vi "Coral Controller.vi"(3 "error in":errorcluster) -> ()   [LabVIEW 2023]
doc: "This VI executes continuously carrying out the current operation and responding to updates or new operations. It will often contain the timing or control code that is difficult to place directly in TeleOp. This VI generally opens all sensors and motors and isolates the rest of the robot code from knowing how the operations are carried out."
uses:
  <vilib>/Rock Robotics/WPI/Framework/Completion Status.ctl
  Coral Setpoints.ctl
  Coral Operations.ctl
  Support Code/Teleop Util/Coral States.ctl
  Support Code/Teleop Util/Scoring Levels.ctl
  <vilib>/Rock Robotics/WPI/ThirdParty/REV Robotics/REVLib/Typedef/Spark MAX Idle Mode.ctl
  <vilib>/Rock Robotics/WPI/ThirdParty/REV Robotics/REVLib/Typedef/SPARK Closed Loop Slot.ctl
  <vilib>/Rock Robotics/SystemInterfaces/DIO/FPGA_DIOChannel.ctl
  <vilib>/Rock Robotics/WPI/ThirdParty/REV Robotics/REVLib/Typedef/Spark MAX Control Type.ctl
  <vilib>/Rock Robotics/WPI/ThirdParty/REV Robotics/REVLib/SubVI/Public/SPARK Open Brushless.vi
  <vilib>/Rock Robotics/WPI/ThirdParty/REV Robotics/REVLib/SubVI/Public/SPARK Configure Basic Idle Mode.vi
  <vilib>/Rock Robotics/WPI/ThirdParty/REV Robotics/REVLib/SubVI/Public/SPARK Configure Basic Inverted.vi
  <vilib>/Rock Robotics/WPI/ThirdParty/REV Robotics/REVLib/SubVI/Public/SPARK Configure Encoder Conversion Factors.vi
  <vilib>/Rock Robotics/WPI/ThirdParty/REV Robotics/REVLib/SubVI/Public/SPARK Configure Limit Switch Reverse.vi
  <vilib>/Rock Robotics/WPI/ThirdParty/REV Robotics/REVLib/SubVI/Public/SPARK Configure Soft Limit Forward.vi
  <vilib>/Rock Robotics/WPI/ThirdParty/REV Robotics/REVLib/SubVI/Public/SPARK Configure Soft Limit Reverse.vi
  <vilib>/Rock Robotics/WPI/ThirdParty/REV Robotics/REVLib/SubVI/Public/SPARK Configure Power Smart Current Limit.vi
  <vilib>/Rock Robotics/WPI/ThirdParty/REV Robotics/REVLib/SubVI/Public/SPARK Configure Closed Loop Miscellaneous.vi
  <vilib>/Rock Robotics/Network Tables/NT Write String.vi
  Framework/Robot Global Data.vi
  <vilib>/Rock Robotics/Network Tables/NT Read Number.vi
  <vilib>/Rock Robotics/WPI/ThirdParty/REV Robotics/REVLib/SubVI/Public/SPARK Get Encoder Status Position.vi
  <vilib>/Rock Robotics/WPI/ThirdParty/REV Robotics/REVLib/SubVI/Public/SPARK Get Device Status Output Current.vi
  <vilib>/Rock Robotics/WPI/ThirdParty/REV Robotics/REVLib/SubVI/Public/SPARK Get Encoder Status Velocity.vi
  <vilib>/Rock Robotics/Network Tables/NT Write Number.vi
  <vilib>/Rock Robotics/WPI/ThirdParty/REV Robotics/REVLib/Typedef/Spark MAX Limit Switch Polarity.ctl
  <vilib>/Rock Robotics/WPI/ThirdParty/REV Robotics/REVLib/SubVI/Public/SPARK Configure Follower Mode From Ref.vi
  <vilib>/Rock Robotics/WPI/ThirdParty/REV Robotics/REVLib/SubVI/Public/SPARK Configure Limit Switch Forward.vi
  <vilib>/Rock Robotics/Network Tables/NT Write Boolean.vi
panel:
  out "Coral Seen":dbl(graph)
  out "Detect DIO2?":bool
  out "Detect DIO1?":bool
  in  "Arbitrary Feed Forward (0)":dbl=0.7
  out "End Time":dbl=1.16
  out "Current":dbl(graph)=8.571428571428571
  in  "Trapezoid Fly off?":bool
  out "Grounded Trapezoid":cluster{"Sensor Velocity":dbl, "Numeric":dbl}[](graph)=[{"Sensor Velocity"=-0.8645192980766296, "Numeric"=0.0}, {"Sensor Velocity"=-0.6395611763000488, "Numeric"=130.0}, {"Sensor Velocity"=0.6042479872703552, "Numeric"=260.0}, {"Sensor Velocity"=9.457396507263184, "Numeric"=390.0}, {"Sensor Velocity"=42.07109451293945, "Numeric"=520.0}, {"Sensor Velocity"=110.76964569091797, "Numeric"=650.0}, {"Sensor Velocity"=199.5862579345703, "Numeric"=780.0}, {"Sensor Velocity"=314.9165344238281, "Numeric"=910.0000000000001}, {"Sensor Velocity"=458.24102783203125, "Numeric"=1040.0}, {"Sensor Velocity"=610.0145263671875, "Numeric"=1170.0}, {"Sensor Velocity"=743.2603759765625, "Numeric"=1300.0}, {"Sensor Velocity"=877.9422607421875, "Numeric"=1430.0}, {"Sensor Velocity"=1007.7548828125, "Numeric"=1560.0}, {"Sensor Velocity"=1120.9271240234375, "Numeric"=1690.0}, {"Sensor Velocity"=1236.4169921875, "Numeric"=1820.0000000000002}, {"Sensor Velocity"=1353.0106201171875, "Numeric"=1950.0}, {"Sensor Velocity"=1475.4154052734375, "Numeric"=2080.0}, {"Sensor Velocity"=1603.7957763671875, "Numeric"=2210.0}, {"Sensor Velocity"=1739.5540771484375, "Numeric"=2340.0}, {"Sensor Velocity"=1868.9521484375, "Numeric"=2470.0}, {"Sensor Velocity"=1992.354736328125, "Numeric"=2600.0}, {"Sensor Velocity"=2117.319091796875, "Numeric"=2730.0}, {"Sensor Velocity"=2234.47900390625, "Numeric"=2860.0}, {"Sensor Velocity"=2350.825439453125, "Numeric"=2990.0}, {"Sensor Velocity"=2471.163818359375, "Numeric"=3120.0}, {"Sensor Velocity"=2591.919189453125, "Numeric"=3250.0}, {"Sensor Velocity"=2712.11083984375, "Numeric"=3380.0}, {"Sensor Velocity"=2833.210205078125, "Numeric"=3510.0000000000005}, {"Sensor Velocity"=2956.64697265625, "Numeric"=3640.0000000000005}, {"Sensor Velocity"=3072.224365234375, "Numeric"=3769.9999999999995}, {"Sensor Velocity"=3190.86376953125, "Numeric"=3810.188567638397}, {"Sensor Velocity"=3313.081298828125, "Numeric"=3680.188567638397}, {"Sensor Velocity"=3434.365234375, "Numeric"=3550.188567638397}, {"Sensor Velocity"=3542.049560546875, "Numeric"=3420.188567638397}, {"Sensor Velocity"=3607.70849609375, "Numeric"=3290.1885676383968}, {"Sensor Velocity"=3606.5849609375, "Numeric"=3160.1885676383977}, {"Sensor Velocity"=3526.638427734375, "Numeric"=3030.188567638397}, {"Sensor Velocity"=3369.229248046875, "Numeric"=2900.188567638397}, {"Sensor Velocity"=3153.94970703125, "Numeric"=2770.188567638397}, {"Sensor Velocity"=2924.535400390625, "Numeric"=2640.188567638397}, {"Sensor Velocity"=2719.2861328125, "Numeric"=2510.188567638397}, {"Sensor Velocity"=2555.581787109375, "Numeric"=2380.188567638397}, {"Sensor Velocity"=2438.929443359375, "Numeric"=2250.188567638397}, {"Sensor Velocity"=2356.54638671875, "Numeric"=2120.188567638397}, {"Sensor Velocity"=2284.232666015625, "Numeric"=1990.1885676383972}, {"Sensor Velocity"=2199.458740234375, "Numeric"=1860.188567638397}, {"Sensor Velocity"=2090.252197265625, "Numeric"=1730.1885676383968}, {"Sensor Velocity"=1953.88427734375, "Numeric"=1600.1885676383977}, {"Sensor Velocity"=1794.5289306640625, "Numeric"=1470.1885676383977}, {"Sensor Velocity"=1637.5787353515625, "Numeric"=1340.1885676383972}, {"Sensor Velocity"=1485.1500244140625, "Numeric"=1210.1885676383972}, {"Sensor Velocity"=1346.7877197265625, "Numeric"=1080.1885676383972}, {"Sensor Velocity"=1225.3587646484375, "Numeric"=950.1885676383968}, {"Sensor Velocity"=1115.109619140625, "Numeric"=820.1885676383968}, {"Sensor Velocity"=999.061279296875, "Numeric"=690.1885676383968}, {"Sensor Velocity"=821.3626708984375, "Numeric"=560.1885676383968}, {"Sensor Velocity"=596.3208618164062, "Numeric"=430.1885676383963}, {"Sensor Velocity"=392.0470886230469, "Numeric"=300.18856763839767}, {"Sensor Velocity"=209.99317932128906, "Numeric"=170.18856763839767}, {"Sensor Velocity"=60.287471771240234, "Numeric"=0.0}, {"Sensor Velocity"=-4.871912956237793, "Numeric"=0.0}]
  out "Sensor Experiment":bool
  out "Post-Trapezoid Sensor Position":dbl=-34.25307083129883
  out "Scoring Sequence Trapezoid":cluster{"Sensor Velocity":dbl, "Numeric":dbl}[](graph)=[{"Sensor Velocity"=0.0, "Numeric"=-0.0}, {"Sensor Velocity"=0.0026157922111451626, "Numeric"=-130.0}, {"Sensor Velocity"=-2.9558451175689697, "Numeric"=-260.0}, {"Sensor Velocity"=-16.448101043701172, "Numeric"=-390.0}, {"Sensor Velocity"=-48.15019607543945, "Numeric"=-520.0}, {"Sensor Velocity"=-107.9851303100586, "Numeric"=-650.0}, {"Sensor Velocity"=-196.86322021484375, "Numeric"=-780.0}, {"Sensor Velocity"=-303.8765869140625, "Numeric"=-910.0000000000001}, {"Sensor Velocity"=-431.81890869140625, "Numeric"=-1040.0}, {"Sensor Velocity"=-570.7528076171875, "Numeric"=-1170.0}, {"Sensor Velocity"=-702.0759887695312, "Numeric"=-1300.0}, {"Sensor Velocity"=-836.3681640625, "Numeric"=-1430.0}, {"Sensor Velocity"=-966.5980224609375, "Numeric"=-1560.0}, {"Sensor Velocity"=-1093.2154541015625, "Numeric"=-1690.0}, {"Sensor Velocity"=-1219.048095703125, "Numeric"=-1820.0000000000002}, {"Sensor Velocity"=-1337.7606201171875, "Numeric"=-1950.0}, {"Sensor Velocity"=-1451.64306640625, "Numeric"=-2080.0}, {"Sensor Velocity"=-1571.863525390625, "Numeric"=-2210.0}, {"Sensor Velocity"=-1691.6943359375, "Numeric"=-2340.0}, {"Sensor Velocity"=-1812.6131591796875, "Numeric"=-2470.0}, {"Sensor Velocity"=-1932.349853515625, "Numeric"=-2600.0}, {"Sensor Velocity"=-2050.272216796875, "Numeric"=-2730.0}, {"Sensor Velocity"=-2164.339111328125, "Numeric"=-2860.0}, {"Sensor Velocity"=-2275.850341796875, "Numeric"=-2990.0}, {"Sensor Velocity"=-2386.736328125, "Numeric"=-3120.0}, {"Sensor Velocity"=-2496.785400390625, "Numeric"=-3250.0}, {"Sensor Velocity"=-2606.660400390625, "Numeric"=-3380.0}, {"Sensor Velocity"=-2717.8173828125, "Numeric"=-3510.0000000000005}, {"Sensor Velocity"=-2827.43994140625, "Numeric"=-3640.0000000000005}, {"Sensor Velocity"=-2936.3876953125, "Numeric"=-3769.9999999999995}, {"Sensor Velocity"=-3045.58251953125, "Numeric"=-3845.9956407546997}, {"Sensor Velocity"=-3152.45458984375, "Numeric"=-3715.9956407546997}, {"Sensor Velocity"=-3255.081298828125, "Numeric"=-3585.9956407546997}, {"Sensor Velocity"=-3346.31103515625, "Numeric"=-3455.9956407546997}, {"Sensor Velocity"=-3405.5927734375, "Numeric"=-3325.9956407546993}, {"Sensor Velocity"=-3413.553955078125, "Numeric"=-3195.9956407547}, {"Sensor Velocity"=-3357.670166015625, "Numeric"=-3065.9956407546997}, {"Sensor Velocity"=-3238.325927734375, "Numeric"=-2935.9956407546997}, {"Sensor Velocity"=-3070.0546875, "Numeric"=-2805.9956407546997}, {"Sensor Velocity"=-2879.5595703125, "Numeric"=-2675.9956407546997}, {"Sensor Velocity"=-2695.614501953125, "Numeric"=-2545.9956407546997}, {"Sensor Velocity"=-2537.822021484375, "Numeric"=-2415.9956407546997}, {"Sensor Velocity"=-2411.872802734375, "Numeric"=-2285.9956407546997}, {"Sensor Velocity"=-2310.73583984375, "Numeric"=-2155.9956407546997}, {"Sensor Velocity"=-2222.242431640625, "Numeric"=-2025.9956407546997}, {"Sensor Velocity"=-2135.021484375, "Numeric"=-1895.9956407546995}, {"Sensor Velocity"=-2037.541259765625, "Numeric"=-1765.9956407546993}, {"Sensor Velocity"=-1922.8583984375, "Numeric"=-1635.9956407547002}, {"Sensor Velocity"=-1792.849609375, "Numeric"=-1505.9956407547002}, {"Sensor Velocity"=-1655.527099609375, "Numeric"=-1375.9956407546997}, {"Sensor Velocity"=-1512.610595703125, "Numeric"=-1245.9956407546997}, {"Sensor Velocity"=-1377.0655517578125, "Numeric"=-1115.9956407546997}, {"Sensor Velocity"=-1248.7752685546875, "Numeric"=-985.9956407546993}, {"Sensor Velocity"=-1129.1943359375, "Numeric"=-855.9956407546993}, {"Sensor Velocity"=-1015.5289916992188, "Numeric"=-725.9956407546993}, {"Sensor Velocity"=-904.607666015625, "Numeric"=-595.9956407546993}, {"Sensor Velocity"=-785.28564453125, "Numeric"=-465.9956407546988}, {"Sensor Velocity"=-665.362060546875, "Numeric"=-335.99564075470016}, {"Sensor Velocity"=-540.5089721679688, "Numeric"=-205.99564075470016}, {"Sensor Velocity"=-408.8169250488281, "Numeric"=-75.99564075470016}, {"Sensor Velocity"=-278.9245300292969, "Numeric"=0.0}, {"Sensor Velocity"=-164.08602905273438, "Numeric"=0.0}]
  in  "Acceleration Max":dbl=6500.0
  in  "Velocity Max":dbl=4400.0
  out "Coral Seen":dbl
  out "Velocity Chart for Tuning":dbl(graph)=794.4134521484375
  in  "Launcher PID":T1={"P Gain"=0.0, "I Gain"=1e-06, "D Gain"=0.0, "F Gain"=0.0001, "I Zone"=0.0, "Min Output"=-0.5, "Max Output"=0.5}
  in  "Max I Accum":dbl=100.0
  in  "L4 PID Constant":T1={"P Gain"=0.0, "I Gain"=0.0, "D Gain"=0.0, "F Gain"=0.0, "I Zone"=0.0, "Min Output"=-0.8, "Max Output"=0.8}
  in  "coral threshold":dbl=25.0
  in  "Distance Decrease Grounded":dbl
  out "Command Timing":u32(graph)=17
  in  "Distance Decrease":dbl
  out "Intake Trapezoid Chart":cluster{"Sensor Velocity":dbl, "Numeric":dbl}[](graph)
  out "Position Chart (All Time)":cluster{"Sensor Position":dbl}(graph)={"Sensor Position"=0.0320870541036129}
  in  "L4 Increased FF":dbl=-0.32
  out "Post Position Correction":dbl=-34.25307083129883
  out "detect?":bool
  in  "sensor speed launcher":dbl=1250.0
  in  "launcher speed":dbl=1250.0
  in  "FF multiplier":dbl=0.39
  out "Pivot Chart":T2(graph)={"Sensor Velocity"=-4.928565979003906, "Arbitrary Feedforward"=-6.429}
  in  "Velocity PID Test":T1={"P Gain"=0.0002, "I Gain"=0.0, "D Gain"=0.0, "F Gain"=0.00015, "I Zone"=0.0, "Min Output"=-1.0, "Max Output"=1.0}
  in  "Positional PID Test":T1={"P Gain"=0.07, "I Gain"=0.0, "D Gain"=0.0, "F Gain"=0.0, "I Zone"=0.0, "Min Output"=-0.6, "Max Output"=0.6}
  in  "Intake Pivot Test":T1={"P Gain"=0.09, "I Gain"=0.0, "D Gain"=0.0, "F Gain"=-0.0, "I Zone"=0.0, "Min Output"=-0.8, "Max Output"=0.8}
  in  "detected speed (0)":dbl
  in  "FeedForward Constants":cluster{"kA":dbl, "kS":dbl, "kG":dbl, "kV":dbl}={"kA"=0.0, "kS"=0.0, "kG"=-0.32, "kV"=0.0}
  in  "intake setpoint":dbl=-0.95
  in  "Interactive Values":T3
  out "Current\nCmd":string="Started at  13:46:20.190\n: Immediate,  CS Grounded, SS Default"
  in  "Buttons":cluster{"Execute Cmd":bool, "Abort Cmd":bool}
  out "Command Timing":cluster{"Start Time (ms)":u32, "Iterations":i32}={"Start Time (ms)"=2495487, "Iterations"=0}
  out "Status":T7=enum."Aborted"
  # "irrelevant for now"
  # "sarah wuz here\nreasonable terms\nriyasonable terms"
  # "luke was here(maybe idk anymore)"
  # "intake speed: must be negative"
  # "launchee speed when intaking"
  # "Interactive Command: You may fill in the settings for a command\nand schedule it with the Execute button. You can observe and abort\nany command while fine tuning the code for the controller."
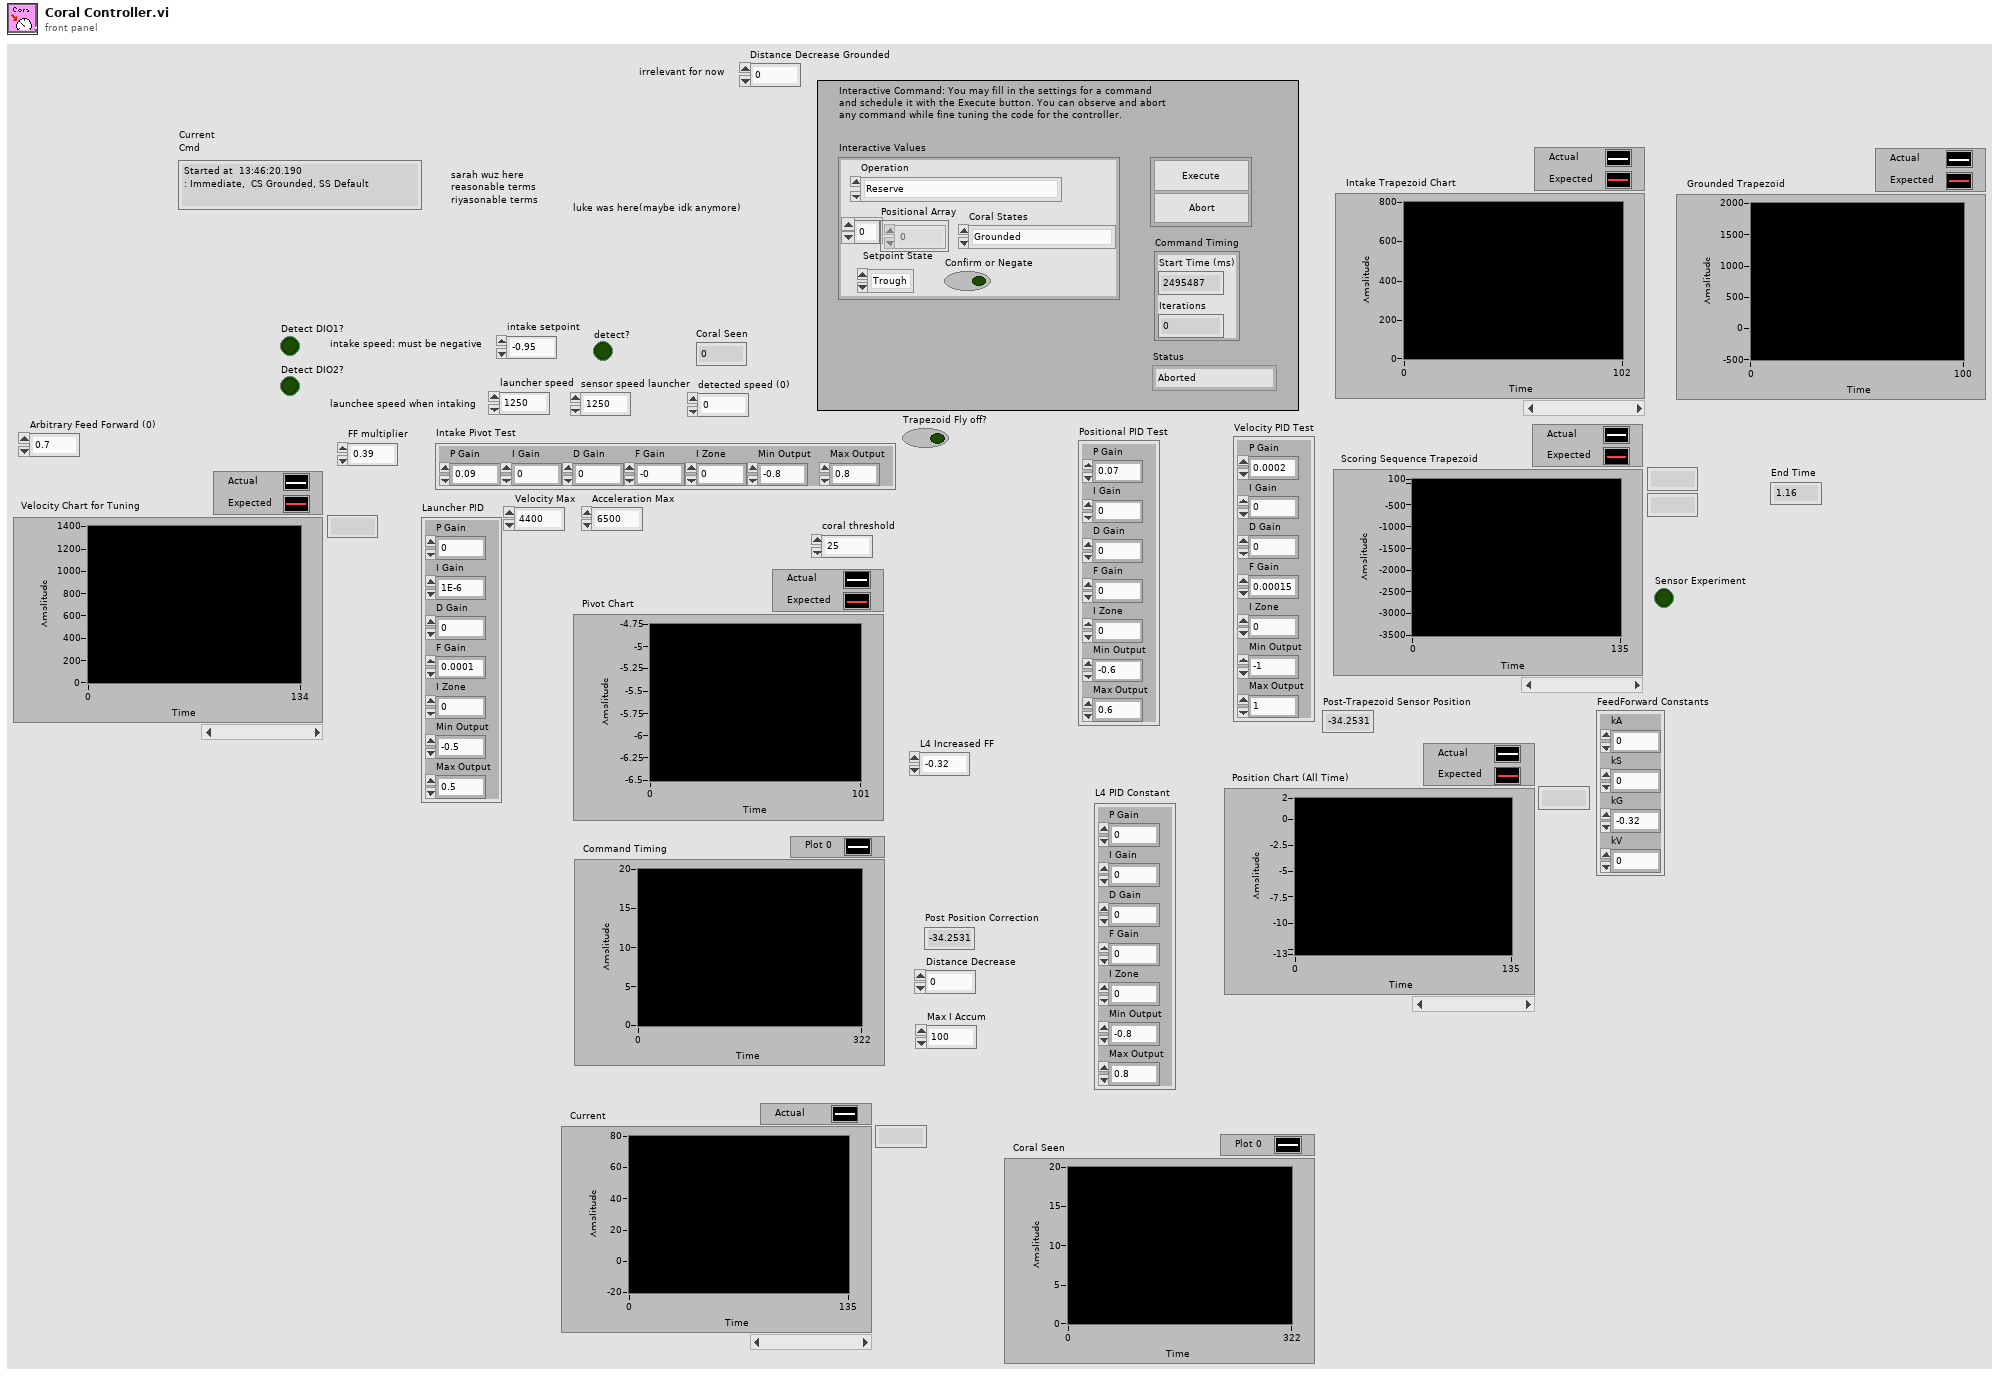
[diagram p1: front panel]
types:
  T1 = cluster{"P Gain":dbl, "I Gain":dbl, "D Gain":dbl, "F Gain":dbl, "I Zone":dbl, "Min Output":dbl, "Max Output":dbl}
  T2 = cluster{"Sensor Velocity":dbl, "Arbitrary Feedforward":dbl}
  T3 = typedef "Coral Setpoints.ctl" = cluster{"Operation":T4, "Coral States":T5, "Confirm or Negate":bool, "Positional Array":dbl[], "Setpoint State":T6}
  T4 = typedef "Coral Operations.ctl" = enum16{"Reserve", "Read Current", "Immediate", "Calibrate"}
  T5 = typedef "Coral States.ctl" = enum16{"Grounded", "Coral Intake", "Scoring Sequence", "Hold Position", "Score", "Manual Override", "Climb Safety Mode"}
  T6 = typedef "Scoring Levels.ctl" = enum16{"Trough", "L2", "L3", "L4", "Default"}
  T7 = typedef "Completion Status.ctl" = enum16{"Successful", "Aborted", "Incomplete"}
  T8 = typedef "FPGA_DIOChannel.ctl" = enum8{"DIO 0", "DIO 1", "DIO 2", "DIO 3", "DIO 4", "DIO 5", "DIO 6", "DIO 7", "DIO 8", "DIO 9", "DIO MXP 0", "DIO MXP 1", "DIO MXP 2", "DIO MXP 3", "DIO MXP 4", "DIO MXP 5", "DIO MXP 6", "DIO MXP 7", "DIO MXP 8", "DIO MXP 9", "DIO MXP 10", "DIO MXP 11", "DIO MXP 12", "DIO MXP 13", "DIO MXP 14", "DIO MXP 15", "SPI Port CS1", "SPI Port CS2", "SPI Port CS3", "SPI Port MISO", "SPI Port MOSI", "Invalid"}
  T9 = typedef "Spark MAX Idle Mode.ctl" = enum16{"Coast", "Brake"}
  T10 = typedef "SPARK Closed Loop Slot.ctl" = u16
  T11 = typedef "WPI_MotorControlDeviceRef.ctl" = cluster{"DeviceStatus":errorcluster, "Type":T12, "PWM":cluster{"PWM Channel":T13, "DeadBand":T14}, "CAN":cluster{"Device Number":u8, "SetOutput VI Ref":variant, "GetOutput VI Ref":variant, "Enable VI Ref":variant, "Disable VI Ref":variant, "Data":variant}, "Invert":bool, "DIO PWM":cluster{"PWM \"Enable\" Channel":T13, "DIOChannel":T8, "PWM Rate":dbl}}
  T12 = typedef "WPI_MotorControlType.ctl" = enum16{"PWM", "CAN", "DIO PWM"}
  T13 = typedef "FPGA_DIOPWMChannel.ctl" = enum8{"PWM 0", "PWM 1", "PWM 2", "PWM 3", "PWM 4", "PWM 5", "PWM 6", "PWM 7", "PWM 8", "PWM 9", "PWM MXP 0", "PWM MXP 1", "PWM MXP 2", "PWM MXP 3", "PWM MXP 4", "PWM MXP 5", "PWM MXP 6", "PWM MXP 7", "PWM MXP 8", "PWM MXP 9", "Invalid"}
  T14 = typedef "WPI_PWMDeadband.ctl" = cluster{"Name":string, "maxPositivePwm":i32, "minPositivePwm":i32, "centerPwm":i32, "maxNegativePwm":i32, "minNegativePwm":i32, "angularRange":u16}
  T15 = typedef "Command Status Info.ctl" = cluster{"Name":string, "Status":T7, "notifier out":T16}
  T16 = typedef "Completion Notifier.ctl" = refnum<notifier>
  T17 = typedef "WPI_DigitalInputDevRef.ctl" = cluster{"DevStatus":errorcluster, "DIO Channel":T8}
  T18 = cluster{"Current Command":T3, "Command Timing":cluster{"Start Time (ms)":u32, "Iterations":i32}, "Command Arguments":cluster{"Command Info":T15, "Description":string, "Default Command":T3, "queue out":refnum<queue>, "Subsystem Name":string}}
  T19 = typedef "Spark MAX Control Type.ctl" = enum16{"Percent VBus", "Voltage", "Velocity", "Position", "Smart Motion", "Current", "Smart Velocity", "MAXMotion Position", "MAXMotion Velocity"}
  T20 = typedef "Spark MAX Limit Switch Polarity.ctl" = enum16{"Normally Open", "Normally Closed"}
  T21 = cluster{"Setpoint Configs":cluster{"Scoring Setpoint":T6, "Position Setpoint":dbl, "Trapezoid":dbl[], "Score Power":dbl}[]}
  T22 = cluster{"Scoring Setpoint":T6, "Position Setpoint":dbl, "Trapezoid":dbl[], "Score Power":dbl}[]
  T23 = cluster{"Scoring Setpoint":T6, "Position Setpoint":dbl, "Trapezoid":dbl[], "Score Power":dbl}
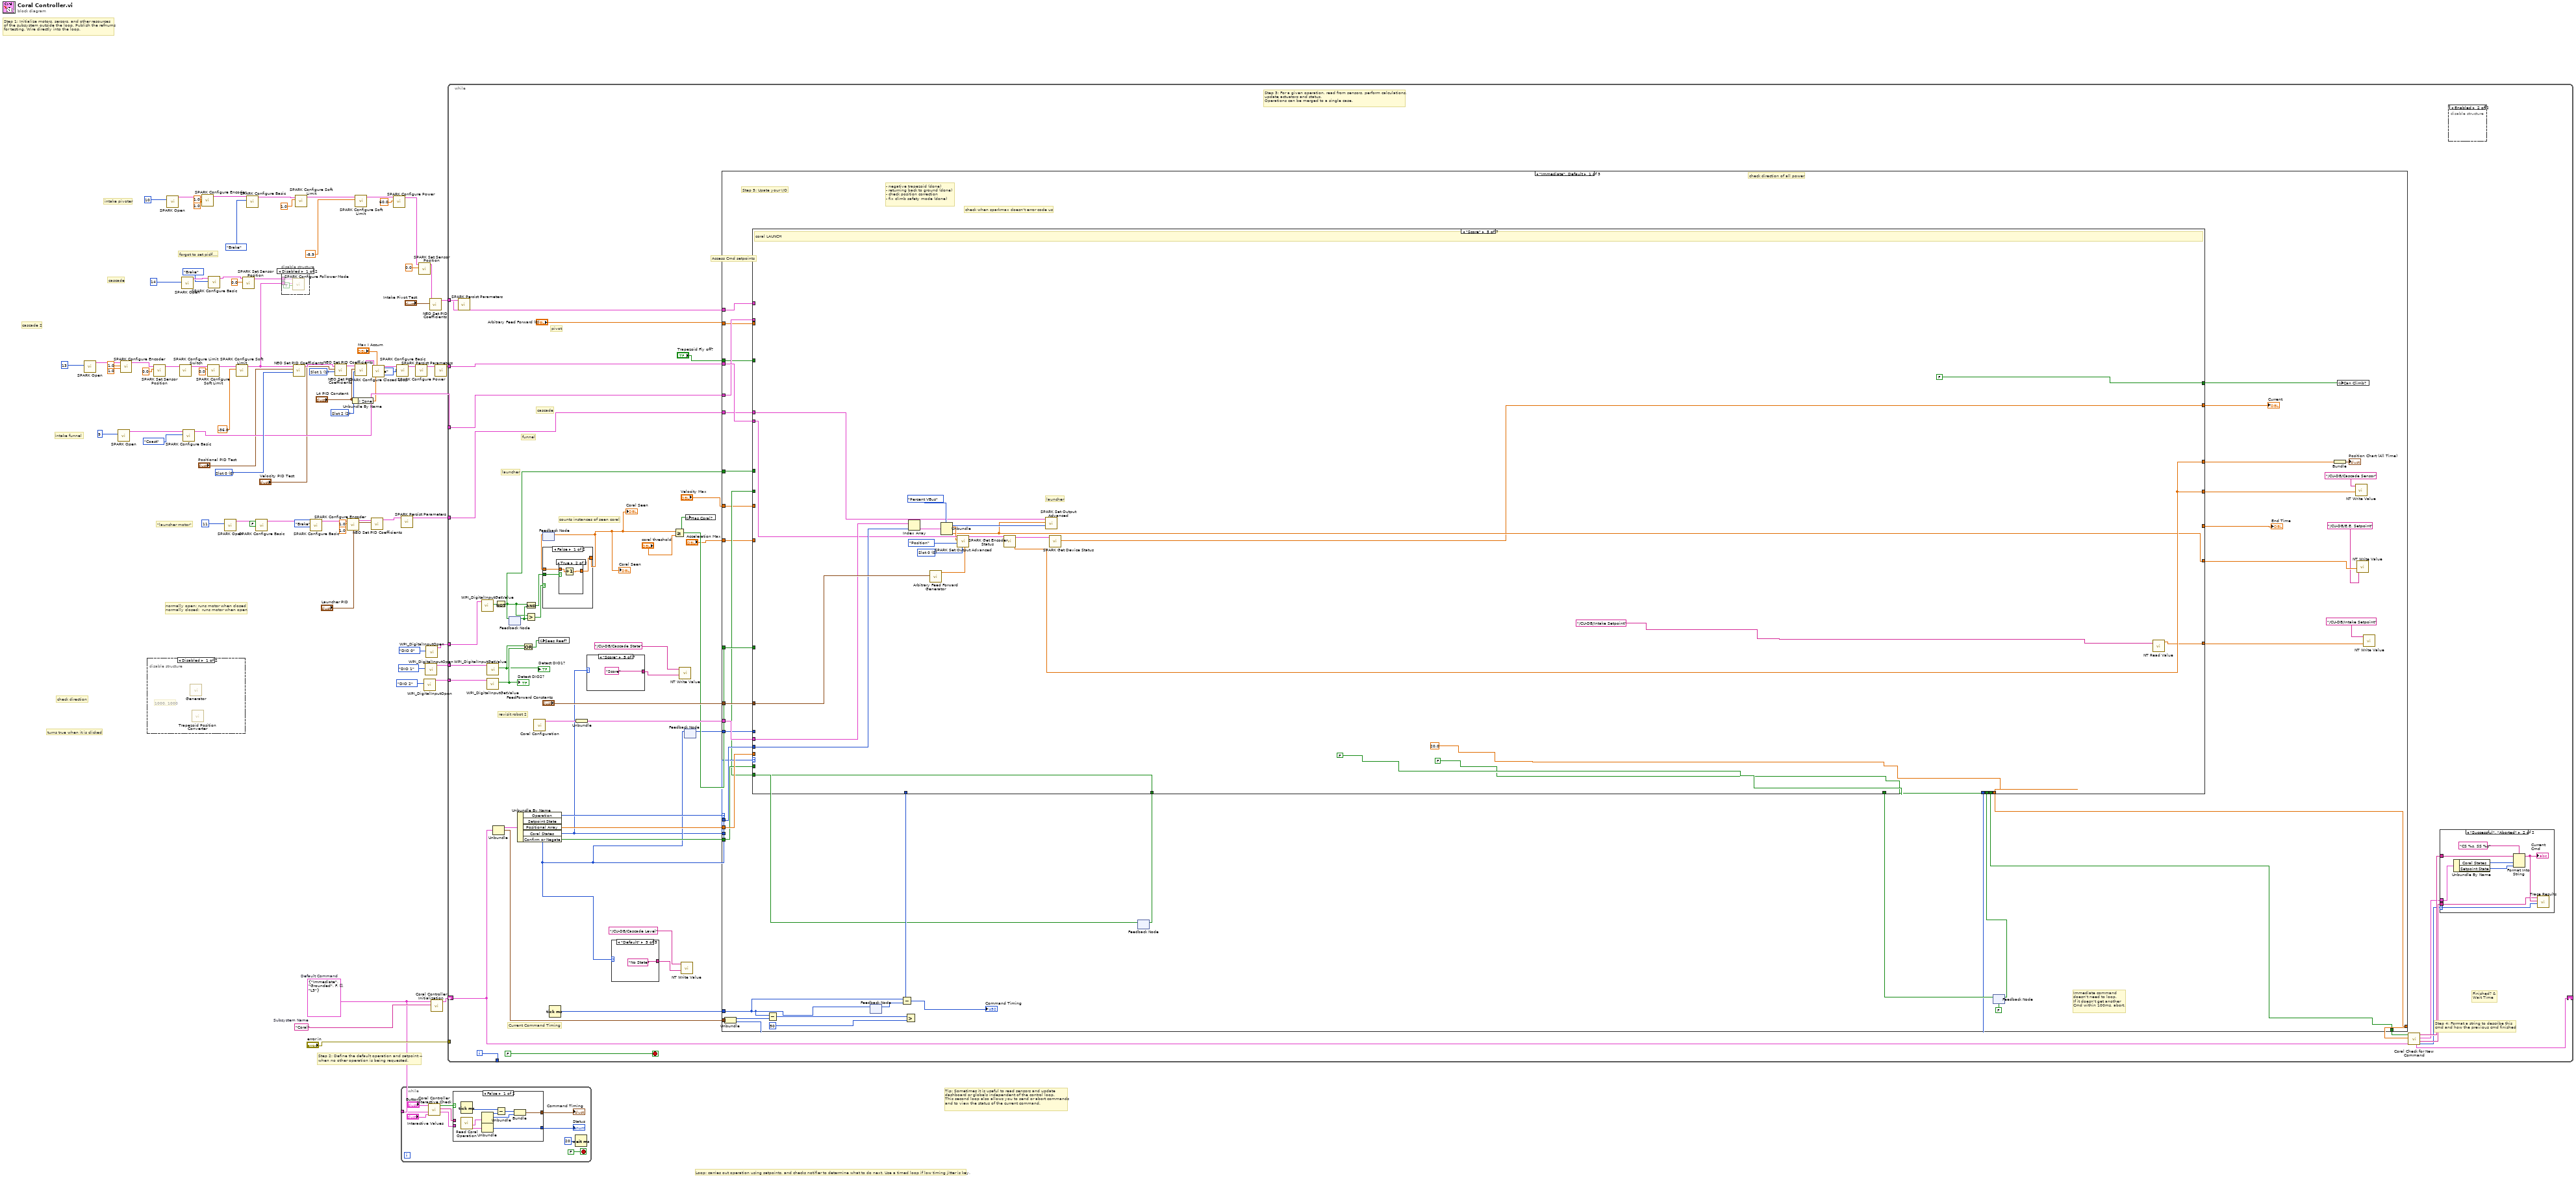
[diagram p0: block diagram]
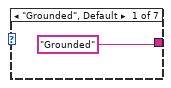
[diagram p2: hidden frame]
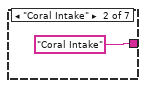
[diagram p3: hidden frame]
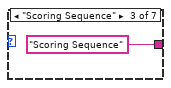
[diagram p4: hidden frame]
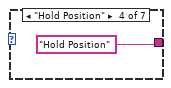
[diagram p5: hidden frame]
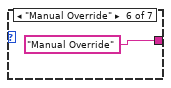
[diagram p6: hidden frame]
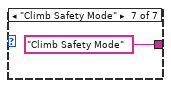
[diagram p7: hidden frame]
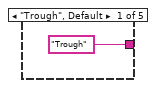
[diagram p8: hidden frame]
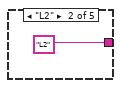
[diagram p9: hidden frame]
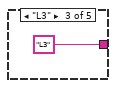
[diagram p10: hidden frame]
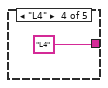
[diagram p11: hidden frame]
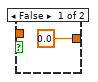
[diagram p12: hidden frame]
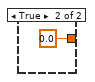
[diagram p13: hidden frame]
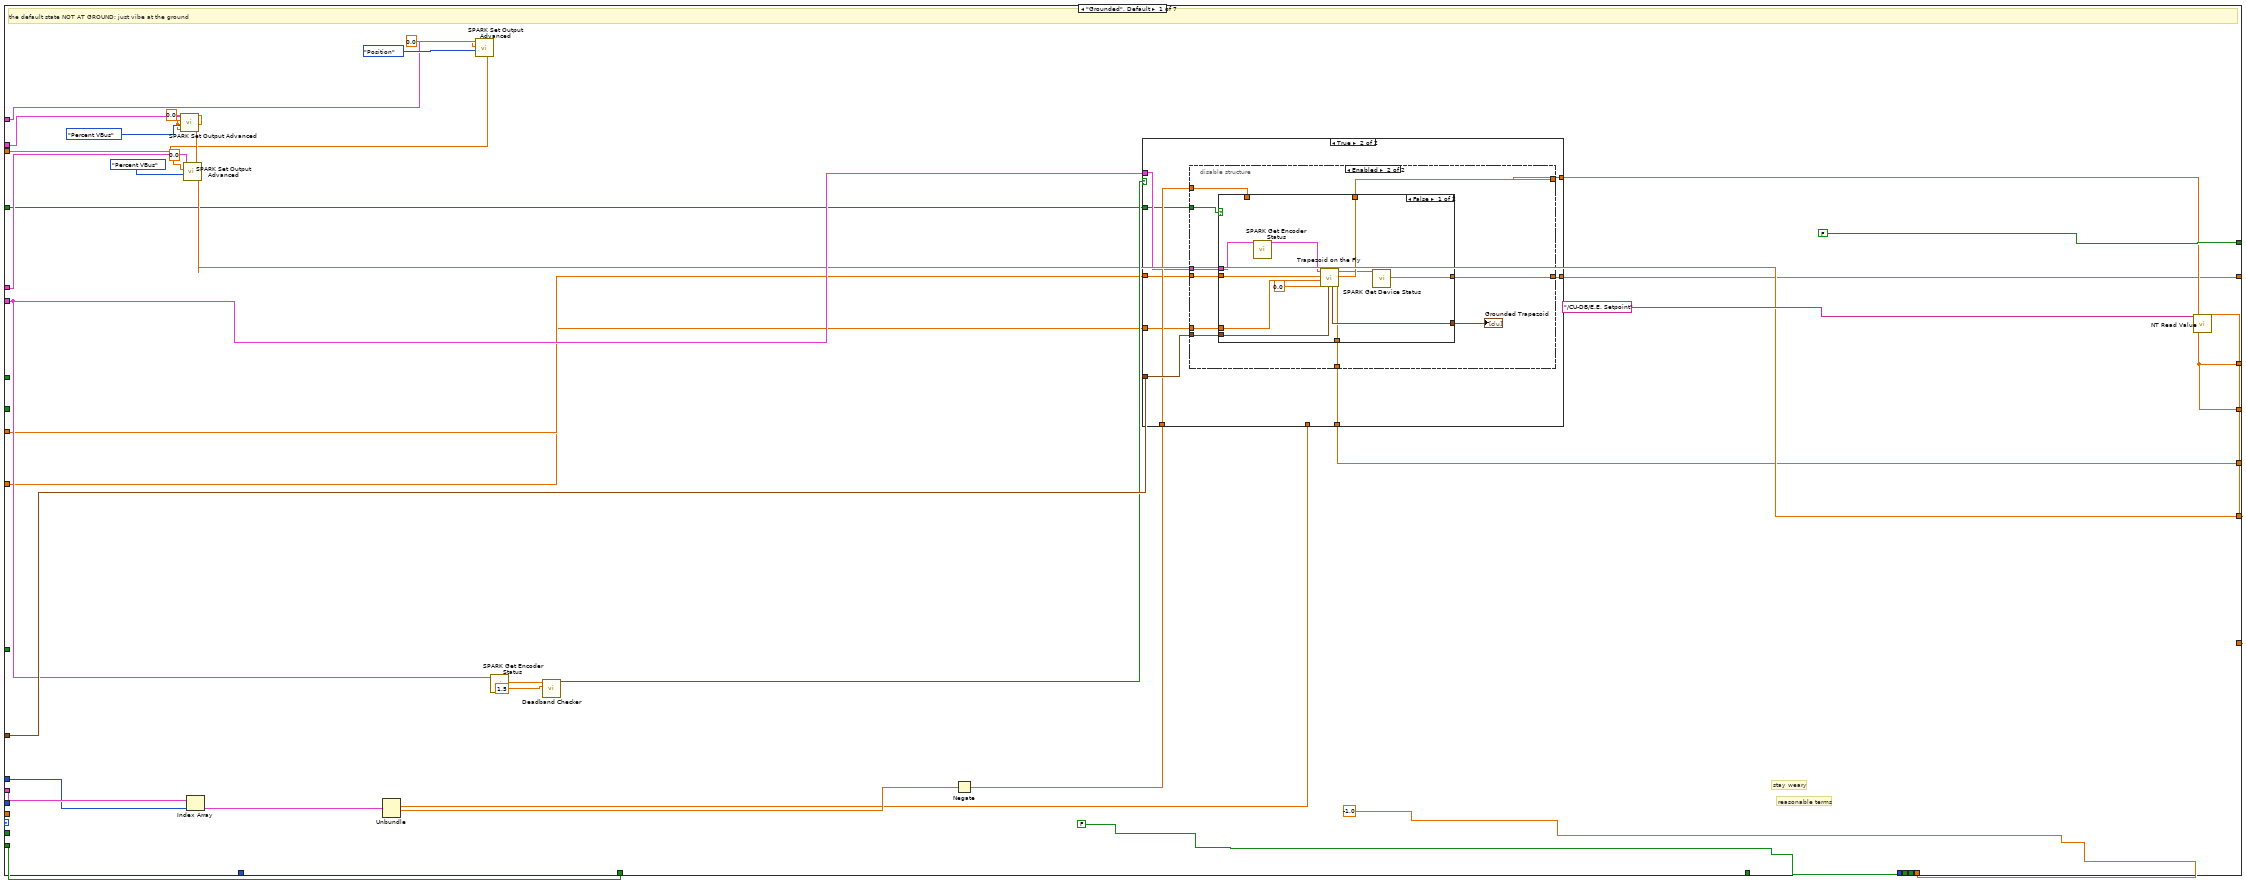
[diagram p14: hidden frame]
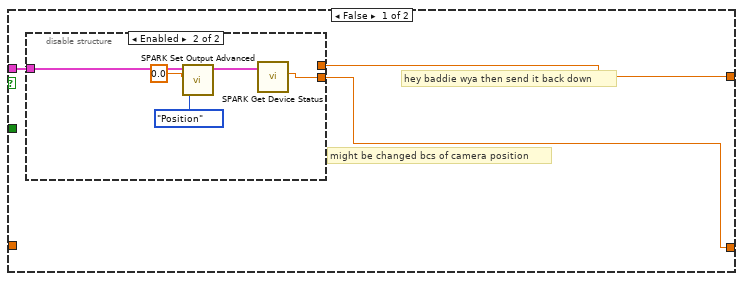
[diagram p15: hidden frame]
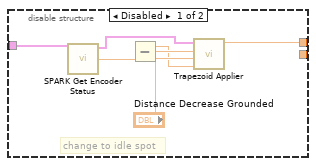
[diagram p16: hidden frame]
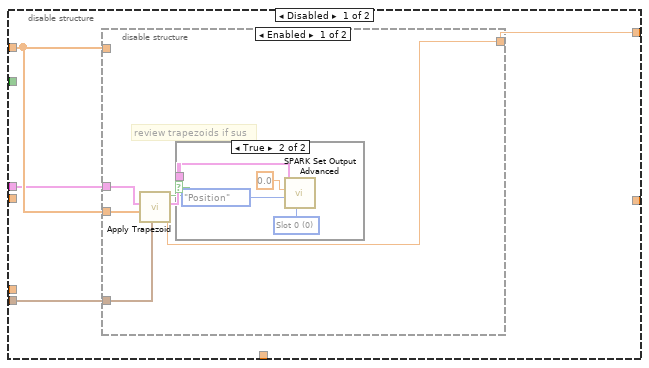
[diagram p17: hidden frame]
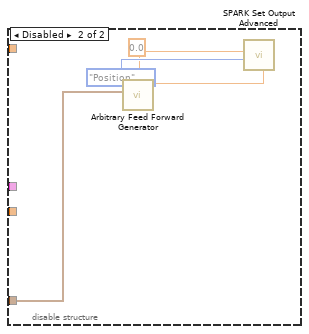
[diagram p19: hidden frame]
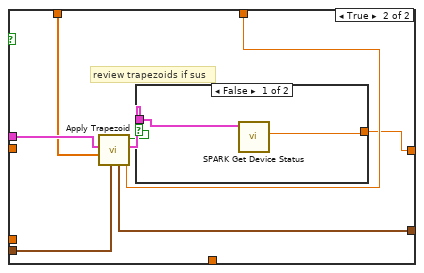
[diagram p20: hidden frame]
diagram:
  (unwired) 1.0 ("Velocity Conversion Factor")
  w18 = T10 2 items=["Slot 0", "Slot 1", "Slot 2", "Slot 3"] ("Loop Slot")
  w58 = T10 1 items=["Slot 0", "Slot 1", "Slot 2", "Slot 3"] ("Loop Slot")
  w60 = T10 0 items=["Slot 0", "Slot 1", "Slot 2", "Slot 3"] ("Loop Slot")
  w74 = T3 {"Operation"=enum."Immediate", "Coral States"=enum."Grounded", "Confirm or Negate"=FALSE, "Positional Array"=[], "Setpoint State"=enum."L3"}  # Default Command
  w75 = "Coral"  # Subsystem Name
  # "intake pivoter"
  # "intake funnel"
  # "cascade 2"
  # "cascade"
  # "turns true when it is clicked"
  # "normally open: runs motor when closed\nnormally closed:  runs motor when open"
  # "check direction"
  # "\"launcher motor\""
  # "forgot to set pidf...."
  # "Tip: Sometimes it is useful to read sensors and update\ndashboard or globals independent of the control loop.\nThis second loop also allows you to send or abort commands\nand to view the status of the current command."
  # "Step 2: Define the default operation and setpoint --\nwhen no other operation is being requested."
  # "Step 1: Initialize motors, sersors, and other resources\nof the subsystem outside the loop. Publish the refnums\nfor testing. Wire directly into the loop."
  # "Loop: carries out operation using setpoints, and checks notifier to determine what to do next. Use a timed loop if low timing jitter is key."
  n1 = call-poly <vilib>:"SPARK Open.vi"("Device Number"=u8 13) -> ("MotorControlDeviceRef"=w68:T11)  [unwired: 9 in, 1 out]
  n2 = call-poly <vilib>:"SPARK Open.vi"("Device Number"=u8 9) -> ("MotorControlDeviceRef"=w50:T11)  [unwired: 9 in, 1 out]
  n3 = call-poly <vilib>:"SPARK Configure Encoder.vi"("Velocity Conversion Factor"=1.0, "Position Conversion Factor"=1.0, "MotorControlDeviceRef in"=w68) -> ("MotorControlDeviceRef out"=w32:T11)  [unwired: 7 in, 1 out]
  n4 = disable-structure shown="Disabled" {
    frame Disabled {
      # "1000, 1000"
      n5 = call "Generator.vi"() -> ("Velocity Max"=w78:dbl, "Acceleration Max"=w79:dbl)  [unwired: 8 in, 2 out]
      n6 = call "Trapezoid Position Converter.vi"() -> ()  [unwired: 11 in, 1 out]
    }
    frame Enabled {
    }
  }
  n7 = call <vilib>:"SPARK Set Sensor Position.vi"("Position"=0.0, "MotorControlDeviceRef"=w32) -> ("MotorControlDeviceRef"=w67:T11)  [unwired: 8 in, 1 out]
  n8 = call-poly <vilib>:"SPARK Open.vi"("Device Number"=u8 10) -> ("MotorControlDeviceRef"=w29:T11)  [unwired: 9 in, 1 out]
  n9 = call-poly <vilib>:"SPARK Configure Limit Switch.vi"("MotorControlDeviceRef in"=w67) -> ("MotorControlDeviceRef out"=w65:T11)  [unwired: 9 in, 1 out]
  n10 = call-poly <vilib>:"SPARK Open.vi"("Device Number"=u8 14) -> ("MotorControlDeviceRef"=w5:T11)  [unwired: 9 in, 1 out]
  n11 = call-poly <vilib>:"SPARK Configure Basic.vi"("Idle Mode"=Spark_MAX_Idle_Mode."Coast", "MotorControlDeviceRef in"=w50) -> ("MotorControlDeviceRef out"=w49:T11)  [unwired: 8 in, 1 out]
  n12 = call-poly <vilib>:"SPARK Configure Encoder.vi"("Velocity Conversion Factor"=1.0, "Position Conversion Factor"=1.0, "MotorControlDeviceRef in"=w29) -> ("MotorControlDeviceRef out"=w28:T11)  [unwired: 7 in, 1 out]
  n13 = call-poly <vilib>:"SPARK Configure Soft Limit.vi"("Soft Limit"=0.0, "MotorControlDeviceRef in"=w65) -> ("MotorControlDeviceRef out"=w71:T11)  [unwired: 8 in, 1 out]
  n14 = call-poly <vilib>:"SPARK Configure Basic.vi"("Idle Mode"=Spark_MAX_Idle_Mode."Brake", "MotorControlDeviceRef in"=w5) -> ("MotorControlDeviceRef out"=w3:T11)  [unwired: 8 in, 1 out]
  n15 = call-poly <vilib>:"SPARK Open.vi"("Device Number"=u8 11) -> ("MotorControlDeviceRef"=w57:T11)  [unwired: 9 in, 1 out]
  n16 = call-poly <vilib>:"SPARK Configure Soft Limit.vi"("Soft Limit"=-36.0, "MotorControlDeviceRef in"=w71) -> ("MotorControlDeviceRef out"=w73:T11)  [unwired: 8 in, 1 out]
  n17 = call <vilib>:"SPARK Set Sensor Position.vi"("Position"=0.0, "MotorControlDeviceRef"=w3) -> ("MotorControlDeviceRef"=w55:T11)  [unwired: 8 in, 1 out]
  n18 = call-poly <vilib>:"SPARK Configure Basic.vi"("Idle Mode"=Spark_MAX_Idle_Mode."Brake", "MotorControlDeviceRef in"=w28) -> ("MotorControlDeviceRef out"=w52:T11)  [unwired: 8 in, 1 out]
  n19 = call-poly <vilib>:"SPARK Configure Basic.vi"("Inverted (F)"=FALSE, "MotorControlDeviceRef in"=w57) -> ("MotorControlDeviceRef out"=w43:T11)  [unwired: 8 in, 1 out]
  n20 = disable-structure shown="Disabled" {
    disable-tunnel: w55 -> [w82 _]
    disable-tunnel: w73 -> [w81 _]
    frame Disabled {
      n21 = call-poly <vilib>:"SPARK Configure Follower Mode.vi"("Invert From Leader"=TRUE, "Leader MotorControlDeviceRef"=w81, "MotorControlDeviceRef in"=w82) -> ()  [unwired: 7 in, 2 out]
    }
    frame Enabled {
    }
  }
  n22 = call "NEO Set PID Coefficients.vi"("Closed Loop Slot"=w60, "PID Constants"="Positional PID Test", "MotorControlDeviceRef in"=w73) -> ("MotorControlDeviceRef out"=w59:T11)  [unwired: 5 in, 1 out]
  n23 = call-poly <vilib>:"SPARK Configure Soft Limit.vi"("Soft Limit"=1.0, "MotorControlDeviceRef in"=w52) -> ("MotorControlDeviceRef out"=w54:T11)  [unwired: 8 in, 1 out]
  n24 = call-poly <vilib>:"SPARK Configure Basic.vi"("Idle Mode"=Spark_MAX_Idle_Mode."Brake", "MotorControlDeviceRef in"=w43) -> ("MotorControlDeviceRef out"=w9:T11)  [unwired: 8 in, 1 out]
  n25 = call "NEO Set PID Coefficients.vi"("Closed Loop Slot"=w58, "PID Constants"="Velocity PID Test", "MotorControlDeviceRef in"=w59) -> ("MotorControlDeviceRef out"=w19:T11)  [unwired: 5 in, 1 out]
  n26 = call-poly <vilib>:"SPARK Configure Encoder.vi"("Position Conversion Factor"=1.0, "MotorControlDeviceRef in"=w9) -> ("MotorControlDeviceRef out"=w8:T11)  [unwired: 8 in, 1 out]
  n27 = Unbundle By Name("L4 PID Constant") -> ("I Zone"=w13:dbl)
  n28 = call-poly <vilib>:"SPARK Configure Soft Limit.vi"("Soft Limit"=-8.9, "MotorControlDeviceRef in"=w54) -> ("MotorControlDeviceRef out"=w51:T11)  [unwired: 8 in, 1 out]
  n29 = call "NEO Set PID Coefficients.vi"("Closed Loop Slot"=w18, "PID Constants"="L4 PID Constant", "MotorControlDeviceRef in"=w19) -> ("MotorControlDeviceRef out"=w17:T11)  [unwired: 5 in, 1 out]
  n30 = call "NEO Set PID Coefficients.vi"("PID Constants"="Launcher PID", "MotorControlDeviceRef in"=w8) -> ("MotorControlDeviceRef out"=w12:T11)  [unwired: 6 in, 1 out]
  n31 = call-poly <vilib>:"SPARK Configure Closed Loop.vi"("Max I Accum"="Max I Accum", "I Zone"=w13, "MotorControlDeviceRef in"=w17) -> ("MotorControlDeviceRef out"=w16:T11)  [unwired: 7 in, 1 out]
  n32 = call-poly <vilib>:"SPARK Configure Power.vi"("Primay Current Limit (80A)"=60.0, "MotorControlDeviceRef in"=w51) -> ("MotorControlDeviceRef out"=w35:T11)  [unwired: 8 in, 1 out]
  n33 = call-poly <vilib>:"SPARK Configure Basic.vi"("Idle Mode"=Spark_MAX_Idle_Mode."Brake", "MotorControlDeviceRef in"=w16) -> ("MotorControlDeviceRef out"=w63:T11)  [unwired: 8 in, 1 out]
  n34 = while {
    tunnel: w74 -> [w89]
    stop <- FALSE stop-if-true
    n35 = call "Coral Controller Interactive Check.vi"("Interactive Command in"="Interactive Values", "Default Command"=w89, "Buttons"="Buttons") -> ("Interactive Command out"=w86:T3, "Trace String"=w87:string, "Schedule"=w88:bool)  [unwired: 6 in]
    n36 = case shown="False" w88 {
      tunnel: [w100 w105] -> w85
      tunnel: w86 -> [_ w103]
      tunnel: [w96 w101] -> w84
      tunnel: w87 -> [_ w104]
      frame False {
        n37 = Tick Count (ms)() -> (millisecond timer value=w95:u32)
        n38 = call "Read Coral Operation.vi"() -> ("Command Info"=w93:T15, "SubSystem Data"=w94:T3)  [unwired: 9 in, 1 out]
        n39 = Unbundle(w94) -> ("Operation"=w99:T4, "Coral States"=w97:T5)  [unwired: 3 out]
        n40 = Unbundle(w93) -> ("Status"=w100:T7)  [unwired: 2 out]
        n41 = Subtract(x=w95, y=w99) -> (x-y=w98:u32)
        n42 = Bundle(w98, "Coral States"=w97) -> (w96:cluster{u32, "Coral States":T5})  [unwired: 1 in]
      }
      frame True {
        n43 = call "Coral Command Helper.vi"("Description"=w104, "SubSystem Data"=w103) -> ("Command Info Out"=w102:T15, "Command Timing"=w101:cluster{"Start Time (ms)":u32, "Iterations":i32})  [unwired: 7 in, 1 out]
        n44 = Unbundle(w102) -> ("Status"=w105:T7)  [unwired: 2 out]
      }
    }
    "Status" <- w85
    "Command Timing" <- w84
    n45 = Wait (ms)(milliseconds to wait=u32 20) -> ()  [unwired: 1 out]
  }
  n46 = call <vilib>:"SPARK Persist Parameters.vi"("MotorControlDeviceRef"=w12) -> ("MotorControlDeviceRef"=w20:T11)  [unwired: 9 in, 1 out]
  n47 = call-poly <vilib>:"SPARK Configure Power.vi"("MotorControlDeviceRef in"=w63) -> ("MotorControlDeviceRef out"=w22:T11)  [unwired: 9 in, 1 out]
  n48 = call <vilib>:"SPARK Set Sensor Position.vi"("Position"=0.0, "MotorControlDeviceRef"=w35) -> ("MotorControlDeviceRef"=w25:T11)  [unwired: 8 in, 1 out]
  n49 = call <vilib>:"WPI_DigitalInputOpen.vi"("DIO Channel"=FPGA_DIOChannel."DIO 2") -> ("DigitalInputDevRef"=w1:T17)  [unwired: 9 in, 1 out]
  n50 = call <vilib>:"WPI_DigitalInputOpen.vi"("DIO Channel"=FPGA_DIOChannel."DIO 1") -> ("DigitalInputDevRef"=w6:T17)  [unwired: 9 in, 1 out]
  n51 = call <vilib>:"WPI_DigitalInputOpen.vi"("DIO Channel"=FPGA_DIOChannel."DIO 0") -> ("DigitalInputDevRef"=w39:T17)  [unwired: 9 in, 1 out]
  n52 = call "NEO Set PID Coefficients.vi"("PID Constants"="Intake Pivot Test", "MotorControlDeviceRef in"=w25) -> ("MotorControlDeviceRef out"=w34:T11)  [unwired: 6 in, 1 out]
  n53 = call "Coral Controller Initialization.vi"("Subsystem Name"=w75, "Default Command"=w74) -> ("Current Command"=w76:T18)  [unwired: 9 in]
  n54 = call <vilib>:"SPARK Persist Parameters.vi"("MotorControlDeviceRef"=w22) -> ("MotorControlDeviceRef"=w21:T11)  [unwired: 9 in, 1 out]
  n55 = call <vilib>:"SPARK Persist Parameters.vi"("MotorControlDeviceRef"=w34) -> ("MotorControlDeviceRef"=w23:T11)  [unwired: 9 in, 1 out]
  n56 = while {
    shift-right: [w147] -> _
    shift-left: w76 -> [w140]
    tunnel: [w153] -> _
    tunnel: "error in" -> [_]
    tunnel: w49 -> [w138]
    tunnel: w20 -> [w139]
    tunnel: w21 -> [w132]
    tunnel: w39 -> [w130]
    tunnel: w23 -> [w133]
    tunnel: w6 -> [w113]
    tunnel: w1 -> [w110]
    i -> [w153]
    stop <- FALSE stop-if-true
    # "counts instances of seen coral"
    # "pivot"
    # "funnel"
    # "cascade"
    # "launcher"
    # "revisit robot 2"
    # "Step 5: Upate your I/O"
    # "Step 4: Format a string to describe this\ncmd and how the previous cmd finished"
    # "Current Command Timing"
    # "Access Cmd setpoints"
    # "Finished? &\nWait Time"
    # "Step 3: For a given operation, read from sensors, perform calculations,\nupdate actuators and status.\nOperations can be merged to a single case."
    n57 = call <vilib>:"WPI_DigitalInputGetValue.vi"("DigitalInputDevRef"=w130) -> ("Value"=w131:bool)  [unwired: 8 in, 2 out]
    n58 = call <vilib>:"WPI_DigitalInputGetValue.vi"("DigitalInputDevRef"=w110) -> ("Value"=w109:bool)  [unwired: 8 in, 2 out]
    "Detect DIO2?" <- w109
    n59 = call <vilib>:"WPI_DigitalInputGetValue.vi"("DigitalInputDevRef"=w113) -> ("Value"=w108:bool)  [unwired: 8 in, 2 out]
    "Detect DIO1?" <- w108
    n60 = Unbundle(w140) -> ("Current Command"=w152:T3, "Command Timing"=w149:cluster{"Start Time (ms)":u32, "Iterations":i32})  [unwired: 1 out]
    n61 = Not(x=w131) -> (.not. x?=w116:bool)
    n62 = feedback-in #1(w116) -> ()
    n63 = feedback #1() -> (w129:bool)  [unwired: 1 in]
    n64 = Unbundle By Name(w152) -> ("Operation"=w151:T4, "Setpoint State"=w120:T6, "Positional Array"=w148:dbl[], "Coral States"=w119:T5, "Confirm or Negate"=w137:bool)
    n65 = Or(x=w108, y=w109) -> (x .or. y?=w107:bool)
    n66 = Greater?(x=w116, y=w129) -> (0:w128:bool)
    n67 = And(x=w116, y=w129) -> (x .and. y?=w126:bool)
    n68 = call "Coral Configuration.vi"() -> ("Coral Config"=w136:T21)  [unwired: 10 in, 1 out]
    n69 = global write "Robot Global Data.vi" "Sees Reef?"(w107) -> ()
    n70 = feedback #2() -> (w127:dbl)  [unwired: 1 in]
    n71 = case shown="False" w128 {
      tunnel: [w167 0.0] -> w106
      tunnel: w127 -> [w168 _]
      tunnel: w126 -> [w169 _]
      frame False {
        n72 = case shown="True" w169 {
          tunnel: w168 -> [_ w172]
          tunnel: [0.0 w171] -> w167
          frame False {
          }
          frame True {
            n73 = Increment(x=w172) -> (x+1=w171:dbl)
          }
        }
      }
      frame True {
      }
    }
    "Coral Seen" <- w106
    "Coral Seen" <- w106
    n74 = feedback-in #2(w106) -> ()
    n75 = Tick Count (ms)() -> (millisecond timer value=w150:u32)
    n76 = Unbundle(w136) -> ("Setpoint Configs"=w134:T22)
    n77 = case shown="\"Score\"" w119 {
      tunnel: ["Grounded" "Coral Intake" "Scoring Sequence" "Hold Position" "Score" "Manual Override" "Climb Safety Mode"] -> w118
      frame "Grounded", Default {
      }
      frame "Coral Intake" {
      }
      frame "Scoring Sequence" {
      }
      frame "Hold Position" {
      }
      frame "Score" {
      }
      frame "Manual Override" {
      }
      frame "Climb Safety Mode" {
      }
    }
    n78 = case shown="\"Default\"" w120 {
      tunnel: ["Trough" "L2" "L3" "L4" "No State"] -> w123
      frame "Trough", Default {
      }
      frame "L2" {
      }
      frame "L3" {
      }
      frame "L4" {
      }
      frame "Default" {
      }
    }
    n79 = Greater Or Equal?(x=w106, y="coral threshold") -> (x >= y?=w124:bool)
    n80 = call-poly <vilib>:"NT Write Value.vi"("value"=w118, "name"="/CU-DB/Cascade State") -> ()  [unwired: 9 in, 1 out]
    n81 = call-poly <vilib>:"NT Write Value.vi"("value"=w123, "name"="/CU-DB/Cascade Level") -> ()  [unwired: 9 in, 1 out]
    n82 = feedback-in #3(w120) -> ()
    n83 = feedback #3() -> (w121:T6)  [unwired: 1 in]
    n84 = global write "Robot Global Data.vi" "Has Coral?"(w124) -> ()
    n85 = case shown="\"Immediate\", Default" w151 {
      tunnel: [w200 -1.0 ("Infinite") w808] -> w145
      tunnel: [w199 FALSE ("ignore previous (F)") FALSE ("ignore previous (F)")] -> w146
      tunnel: w149 -> [w213 _ _]
      tunnel: w120 -> [w206 _ _]
      tunnel: w150 -> [w191 _ _]
      tunnel: w148 -> [w210 _ _]
      tunnel: w119 -> [w205 _ _]
      tunnel: w132 -> [w212 w792 w803]
      tunnel: w139 -> [w211 w783 w802]
      tunnel: w138 -> [w208 w786 w797]
      tunnel: w137 -> [w209 _ _]
      tunnel: w133 -> [w207 w787 w793]
      tunnel: "FeedForward Constants" -> [w204 _ _]
      tunnel: w134 -> [w198 _ _]
      tunnel: w124 -> [w193 _ _]
      tunnel: w121 -> [w189 _ _]
      tunnel: w116 -> [w182 _ _]
      tunnel: "Velocity Max" -> [w179 _ _]
      tunnel: "Acceleration Max" -> [w178 _ _]
      tunnel: "Trapezoid Fly off?" -> [w177 _ _]
      tunnel: "Arbitrary Feed Forward (0)" -> [w174 _ _]
      frame "Immediate", Default {
        # "- negative trapezoid (done)\n- returning back to ground (done)\n- check position correction\n- fix climb safety mode (done)"
        # "check when sparkmax doesn't error code us"
        # "check direction of all power"
        # "Immediate command\ndoesn't need to loop.\nIf it doesn't get another\nCmd within 100ms, abort."
        n86 = Unbundle(w213) -> ("Start Time (ms)"=w216:u32, "Iterations"=w190:i32)
        n87 = Subtract(x=w191, y=w216) -> (x-y=w215:u32)
        n88 = feedback-in #4(w191) -> ()
        n89 = feedback #4() -> (w195:u32)  [unwired: 1 in]
        n90 = Subtract(x=w191, y=w195) -> (x-y=→"Command Timing":u32)
        n91 = Greater?(x=w215, y=u8 50 ("Left Motor")) -> ()  [unwired: 1 out]
        n92 = feedback #5() -> (w180:bool)  [unwired: 1 in]
        n93 = feedback #6(FALSE) -> (w201:bool)
        n94 = case shown="\"Score\"" w205 {
          tunnel: w212 -> [w234 w361 w409 w624 w714 w745 w779]
          tunnel: w211 -> [w247 w347 w413 w626 w711 _ _]
          tunnel: w210 -> [_ _ _ _ _ _ _]
          tunnel: w209 -> [_ _ _ _ _ w744 _]
          tunnel: w206 -> [_ _ _ w613 w716 _ w764]
          tunnel: w198 -> [w239 _ w393 w612 w717 _ w765]
          tunnel: w208 -> [w249 w345 w417 w629 _ _ _]
          tunnel: w207 -> [w244 w344 w416 w620 _ _ w778]
          tunnel: w204 -> [w242 w332 w389 w623 w721 w741 w776]
          tunnel: [FALSE ("Boolean") FALSE ("Boolean") FALSE ("Boolean") FALSE ("Boolean") FALSE ("Boolean") FALSE ("Boolean") FALSE ("Boolean")] -> w199
          tunnel: [FALSE w350 FALSE FALSE FALSE FALSE FALSE] -> w203
          tunnel: [w241 w349 w412 w619 FALSE w739 w772] -> w202
          tunnel: w201 -> [w241 w349 w411 w619 _ w739 w772]
          tunnel: [-1.0 ("Infinite") 20.0 ("Infinite") w400 20.0 ("Infinite") 20.0 ("Infinite") 20.0 ("Infinite") 20.0 ("Infinite")] -> w200
          tunnel: [w228 0.0 w396 w609 w708 w732 w759] -> w197
          tunnel: w193 -> [_ _ w401 _ _ _ _]
          tunnel: w191 -> [_ _ _ _ _ _ _]
          tunnel: w190 -> [_ _ _ _ _ _ _]
          tunnel: w189 -> [w229 _ _ w603 _ _ _]
          tunnel: [w228 nan w396 w609 w708 w732 w759] -> w187
          tunnel: [w226 w338 w395 w607 w707 w730 w757] -> w186
          tunnel: [w225 w340 w394 0.0 w705 w728 w755] -> w183
          tunnel: w182 -> [_ _ _ w587 _ _ w754]
          tunnel: [w224 w339 w388 w586 w704 TRUE w751] -> w181
          tunnel: w180 -> [_ _ _ _ _ _ w752]
          tunnel: w180 -> [w224 w339 w388 _ w704 _ w751]
          tunnel: w179 -> [w223 w334 w387 w594 _ _ _]
          tunnel: w178 -> [w222 w335 w386 w595 _ _ _]
          tunnel: w177 -> [w220 _ w385 w592 _ _ _]
          tunnel: [w219 w336 w382 w590 w702 w725 w749] -> w176
          tunnel: [w218 _ w381 w589 _ _ _] -> w175
          tunnel: w174 -> [w217 _ w380 w588 _ _ w748]
          frame "Grounded", Default {
            w225 = 0.0 ("Setpoint")
            # "reasonable terms"
            # "stay weary"
            # "the default state NOT AT GROUND; just vibe at the ground"
            n95 = call <vilib>:"SPARK Set Output Advanced.vi"("Control Mode"=Spark_MAX_Control_Type."Percent VBus", "Setpoint"=w225, "MotorControlDevRef"=w249) -> ()  [unwired: 7 in, 2 out]
            n96 = call <vilib>:"SPARK Set Output Advanced.vi"("Control Mode"=Spark_MAX_Control_Type."Percent VBus", "Setpoint"=0.0, "MotorControlDevRef"=w247) -> ()  [unwired: 7 in, 2 out]
            n97 = Index Array(array=w239, index=w229) -> (element=w238:T23)
            n98 = Unbundle(w238) -> ("Position Setpoint"=w221:dbl, "Trapezoid"=w230:dbl[])  [unwired: 2 out]
            n99 = call <vilib>:"SPARK Set Output Advanced.vi"("Arbitrary Feed Forward (0)"=w217, "Control Mode"=Spark_MAX_Control_Type."Position", "Setpoint"=0.0 ("t"), "MotorControlDevRef"=w244) -> ()  [unwired: 6 in, 2 out]
            n100 = call-poly <vilib>:"SPARK Get Encoder Status.vi"("MotorControlDevRef in"=w234) -> ("Sensor Position"=w232:dbl)  [unwired: 7 in, 3 out]
            n101 = call "Deadband Checker.vi"("Limit"=1.5, "Value"=w232) -> ("Outside Deadband?"=w233:bool)  [unwired: 9 in]
            n102 = Negate(x=w230) -> (-x=w243:dbl[])
            n103 = case shown="True" w233 {
              tunnel: w234 -> [w252 w272]
              tunnel: w243 -> [_ w273]
              tunnel: w242 -> [_ w274]
              tunnel: [w253 w271] -> w228
              tunnel: w223 -> [_ w270]
              tunnel: w222 -> [_ w269]
              tunnel: w221 -> [_ _]
              tunnel: w220 -> [_ w268]
              tunnel: [w251 w267] -> w219
              tunnel: [_ w266] -> w218
              frame False {
                # "might be changed bcs of camera position"
                # "hey baddie wya then send it back down"
                n104 = disable-structure shown="Enabled" {
                  disable-tunnel: [w260 _] -> w253
                  disable-tunnel: w252 -> [w259 w265]
                  disable-tunnel: [_ w261] -> w251
                  frame Disabled {
                    # "change to idle spot"
                    n105 = call-poly <vilib>:"SPARK Get Encoder Status.vi"("MotorControlDevRef in"=w259) -> ("Sensor Position"=w258:dbl, "MotorControlDevRef out"=w256:T11)  [unwired: 7 in, 2 out]
                    n106 = Subtract(x=w254, y=w258) -> (x-y=w257:dbl)
                    n107 = call "Trapezoid Applier.vi"("Distance Decrease"="Distance Decrease Grounded", "Distance to Setpoint"=w257, "MotorControlDevRef in"=w256) -> ("Sensor Position out"=w260:dbl, "Intended Position"=w254:dbl)  [unwired: 6 in, 1 out]
                  }
                  frame Enabled {
                    n108 = call <vilib>:"SPARK Set Output Advanced.vi"("Control Mode"=Spark_MAX_Control_Type."Position", "Setpoint"=0.0, "MotorControlDevRef"=w265) -> ("MotorControlDevRef"=w262:T11)  [unwired: 7 in, 1 out]
                    n109 = call-poly <vilib>:"SPARK Get Device Status.vi"("MotorControlDevRef in"=w262) -> ("Current"=w261:dbl)  [unwired: 7 in, 3 out]
                  }
                }
              }
              frame True {
                n110 = disable-structure shown="Enabled" {
                  disable-tunnel: w274 -> [w278 w302]
                  disable-tunnel: w273 -> [w277 w299]
                  disable-tunnel: w272 -> [w276 w300]
                  disable-tunnel: [w275 w301] -> w271
                  disable-tunnel: w270 -> [_ w304]
                  disable-tunnel: w269 -> [_ w303]
                  disable-tunnel: w268 -> [_ w298]
                  disable-tunnel: [_ w297] -> w267
                  disable-tunnel: [_ w295] -> w266
                  frame Disabled {
                    n111 = disable-structure shown="Enabled" {
                      disable-tunnel: w277 -> [_ _]
                      disable-tunnel: w278 -> [w285 w291]
                      disable-tunnel: w277 -> [w283 _]
                      disable-tunnel: w276 -> [w282 _]
                      disable-tunnel: [w281 _] -> w275
                      frame Enabled {
                        # "review trapezoids if sus"
                        n112 = call "Apply Trapezoid.vi"("FeedForward Constants"=w285, "Velocity values"=w283, "MotorControlDeviceRef in"=w282) -> ("Sensor Position"=w281:dbl, "MotorControlDevRef out"=w280:T11, "Boolean"=w279:bool, "charted V"=w284:cluster{"Sensor Velocity":dbl, "Numeric":dbl}[])  [unwired: 5 in]
                        n113 = case shown="True" w279 {
                          tunnel: w280 -> [_ w289]
                          frame False {
                          }
                          frame True {
                            w286 = T10 0 items=["Slot 0", "Slot 1", "Slot 2", "Slot 3"] ("Closed Loop Slot")
                            n114 = call <vilib>:"SPARK Set Output Advanced.vi"("Closed Loop Slot"=w286, "Control Mode"=Spark_MAX_Control_Type."Position", "Setpoint"=0.0, "MotorControlDevRef"=w289) -> ()  [unwired: 6 in, 2 out]
                          }
                        }
                      }
                      frame Disabled {
                        w290 = 0.0 ("Setpoint")
                        n115 = call "Arbitrary Feed Forward Generator.vi"("Feed Forward Constants"=w291, "Setpoint"=w290) -> ("Arbitrary Feedforward"=w292:dbl)  [unwired: 9 in]
                        n116 = call <vilib>:"SPARK Set Output Advanced.vi"("Arbitrary Feed Forward (0)"=w292, "Control Mode"=Spark_MAX_Control_Type."Position", "Setpoint"=w290) -> ("MotorControlDevRef"=w293:T11)  [unwired: 6 in, 2 out]
                      }
                    }
                  }
                  frame Enabled {
                    n117 = case shown="False" w298 {
                      tunnel: w304 -> [w315 _]
                      tunnel: w303 -> [w314 _]
                      tunnel: w302 -> [w313 w318]
                      tunnel: [w312 w321] -> w301
                      tunnel: w300 -> [w309 w320]
                      tunnel: w299 -> [_ w319]
                      tunnel: [w307 w317] -> w297
                      tunnel: [w306 w316] -> w296
                      tunnel: [w305 _] -> w295
                      frame False {
                        n118 = call-poly <vilib>:"SPARK Get Encoder Status.vi"("MotorControlDevRef in"=w309) -> ("MotorControlDevRef out"=w311:T11)  [unwired: 7 in, 3 out]
                        n119 = call "Trapezoid on the Fly.vi"("FeedForward Constants"=w313, "Setpoint"=0.0 ("x"), "Acceleration Max"=w314, "Velocity Max"=w315, "MotorControlDevRef in"=w311) -> ("End Time"=w305:dbl, "Sensor Position"=w312:dbl, "MotorControlDevRef out"=w308:T11, "charted V"=w306:cluster{"Sensor Velocity":dbl, "Numeric":dbl}[])  [unwired: 1 out]
                        n120 = call-poly <vilib>:"SPARK Get Device Status.vi"("MotorControlDevRef in"=w308) -> ("Current"=w307:dbl)  [unwired: 7 in, 3 out]
                      }
                      frame True {
                        # "review trapezoids if sus"
                        n121 = call "Apply Trapezoid.vi"("FeedForward Constants"=w318, "Velocity values"=w319, "MotorControlDeviceRef in"=w320) -> ("Sensor Position"=w321:dbl, "MotorControlDevRef out"=w323:T11, "Boolean"=w322:bool, "charted V"=w316:cluster{"Sensor Velocity":dbl, "Numeric":dbl}[])  [unwired: 5 in]
                        n122 = case shown="False" w322 {
                          tunnel: w323 -> [w325 w331]
                          tunnel: [w324 w326] -> w317
                          frame False {
                            n123 = call-poly <vilib>:"SPARK Get Device Status.vi"("MotorControlDevRef in"=w325) -> ("Current"=w324:dbl)  [unwired: 7 in, 3 out]
                          }
                          frame True {
                            w328 = T10 0 items=["Slot 0", "Slot 1", "Slot 2", "Slot 3"] ("Closed Loop Slot")
                            n124 = call <vilib>:"SPARK Set Output Advanced.vi"("Closed Loop Slot"=w328, "Control Mode"=Spark_MAX_Control_Type."Position", "Setpoint"=0.0, "MotorControlDevRef"=w331) -> ("MotorControlDevRef"=w327:T11)  [unwired: 6 in, 1 out]
                            n125 = call-poly <vilib>:"SPARK Get Device Status.vi"("MotorControlDevRef in"=w327) -> ("Current"=w326:dbl)  [unwired: 7 in, 3 out]
                          }
                        }
                      }
                    }
                    "Grounded Trapezoid" <- w296
                  }
                }
              }
            }
            n126 = call-poly <vilib>:"NT Read Value.vi"("name"="/CU-DB/E.E. Setpoint") -> ("value"=w226:dbl)  [unwired: 8 in, 2 out]
          }
          frame "Climb Safety Mode" {
            w358 = -6.429 ("Setpoint")
            w338 = 0.0 ("Setpoint")
            w340 = 0.0 ("Setpoint")
            # "pivot intake out of the way and do not move any motors on intake so we do not crash into climb"
            n127 = disable-structure shown="Enabled" {
              disable-tunnel: w361 -> [w363 w374]
              disable-tunnel: w335 -> [_ w369]
              disable-tunnel: w334 -> [_ w368]
              disable-tunnel: 0.0 ("Setpoint") -> [_ w367]
              disable-tunnel: w332 -> [_ w366]
              frame Enabled {
                n128 = call <vilib>:"SPARK Set Output Advanced.vi"("Control Mode"=Spark_MAX_Control_Type."Percent VBus", "Setpoint"=0.0, "MotorControlDevRef"=w363) -> ()  [unwired: 7 in, 2 out]
              }
              frame Disabled {
                n129 = call-poly <vilib>:"SPARK Get Encoder Status.vi"("MotorControlDevRef in"=w374) -> ("Sensor Position"=w370:dbl, "MotorControlDevRef out"=w373:T11)  [unwired: 7 in, 2 out]
                n130 = call "Deadband Checker.vi"("Limit"=1.5, "Value"=w370) -> ("Outside Deadband?"=w371:bool)  [unwired: 9 in]
                n131 = case shown="True" w371 {
                  tunnel: w373 -> [_ w379]
                  tunnel: w369 -> [_ w378]
                  tunnel: w368 -> [_ w377]
                  tunnel: w367 -> [_ w376]
                  tunnel: w366 -> [_ w375]
                  frame False {
                  }
                  frame True {
                    n132 = call "Trapezoid on the Fly.vi"("FeedForward Constants"=w375, "Setpoint"=w376, "Acceleration Max"=w378, "Velocity Max"=w377, "MotorControlDevRef in"=w379) -> ()  [unwired: 5 out]
                  }
                }
              }
            }
            n133 = call <vilib>:"SPARK Set Output Advanced.vi"("Control Mode"=Spark_MAX_Control_Type."Percent VBus", "Setpoint"=w338, "MotorControlDevRef"=w347) -> ("MotorControlDevRef"=w337:T11)  [unwired: 7 in, 1 out]
            n134 = call-poly <vilib>:"SPARK Get Encoder Status.vi"("MotorControlDevRef in"=w344) -> ("Sensor Position"=w352:dbl, "MotorControlDevRef out"=w343:T11)  [unwired: 7 in, 2 out]
            n135 = call-poly <vilib>:"SPARK Get Device Status.vi"("MotorControlDevRef in"=w337) -> ("Current"=w336:dbl)  [unwired: 7 in, 3 out]
            n136 = Less?(x=w352, y=-6.0) -> (x < y?=w350:bool)
            n137 = Divide(x=w352, y=-8.857) -> (x/y=w355:dbl)
            n138 = Bundle("Sensor Position"=w352, "Setpoint"=w358) -> (→"Pivot Chart":cluster{"Sensor Position":dbl, "Setpoint":dbl})  [unwired: 1 in]
            n139 = Multiply(x=w355, y="FF multiplier") -> (x*y=w353:dbl)
            n140 = call <vilib>:"SPARK Set Output Advanced.vi"("Arbitrary Feed Forward (0)"=w353, "Control Mode"=Spark_MAX_Control_Type."Position", "Setpoint"=w358, "MotorControlDevRef"=w343) -> ()  [unwired: 6 in, 2 out]
            n141 = call <vilib>:"SPARK Set Output Advanced.vi"("Control Mode"=Spark_MAX_Control_Type."Percent VBus", "Setpoint"=w340, "MotorControlDevRef"=w345) -> ()  [unwired: 7 in, 2 out]
          }
          frame "Coral Intake" {
            # "changed here"
            # "launcher"
            # "funnel"
            # "trapezoid down if we are not at home (0)"
            # "get cascade position"
            # "pivot"
            # "intake until we reach limit switch then launch coral"
            n142 = call-poly <vilib>:"SPARK Get Encoder Status.vi"("MotorControlDevRef in"=w409) -> ("Sensor Position"=w398:dbl, "MotorControlDevRef out"=w408:T11)  [unwired: 7 in, 2 out]
            n143 = call <vilib>:"SPARK Set Output Advanced.vi"("Arbitrary Feed Forward (0)"=w380, "Control Mode"=Spark_MAX_Control_Type."Position", "Setpoint"=0.0, "MotorControlDevRef"=w416) -> ()  [unwired: 6 in, 2 out]
            n144 = call "Deadband Checker.vi"("Limit"=0.9, "Value"=w398) -> ("Outside Deadband?"=w404:bool)  [unwired: 9 in]
            n145 = Index Array(array=w393) -> (element=w391:T23)  [unwired: 1 in]
            n146 = Unbundle(w391) -> ("Trapezoid"=w390:dbl[])  [unwired: 3 out]
            n147 = case shown="True" w404 {
              tunnel: w408 -> [w420 w461]
              tunnel: [w421 w460] -> w396
              tunnel: w398 -> [w421 w459]
              tunnel: "Distance Decrease" -> [_ w458]
              tunnel: [_ w456] -> w392
              tunnel: w390 -> [_ w457]
              tunnel: w389 -> [w419 w455]
              tunnel: w387 -> [_ w454]
              tunnel: w386 -> [_ w453]
              tunnel: w385 -> [_ w451]
              tunnel: [w418 w450] -> w383
              tunnel: [_ w449] -> w381
              frame False {
                n148 = disable-structure shown="Enabled" {
                  disable-tunnel: w420 -> [w424 w446]
                  disable-tunnel: w419 -> [w422 _]
                  disable-tunnel: [_ w445] -> w418
                  frame Disabled {
                    # "changed here"
                    n149 = call <vilib>:"SPARK Set Output Advanced.vi"("Control Mode"=Spark_MAX_Control_Type."Position", "Setpoint"=0.0, "MotorControlDevRef"=w424) -> ("MotorControlDevRef"=w423:T11)  [unwired: 7 in, 1 out]
                    n150 = disable-structure shown="Enabled" {
                      disable-tunnel: w423 -> [w434 _]
                      disable-tunnel: [w427 _] -> _
                      disable-tunnel: w422 -> [w427 _]
                      frame Enabled {
                        w429 = 0.0 ("Setpoint")
                        n151 = for {
                          N: 1 -> [_]
                          tunnel: [w443] -> w436
                          tunnel: w427 -> [w440]
                          shift-right: [w442] -> w435
                          shift-left: w434 -> [w441]
                          w439 = -0.05 ("Setpoint")
                          (unwired) 0.0 ("Position")
                          n152 = call "Arbitrary Feed Forward Generator.vi"("Feed Forward Constants"=w440, "Setpoint"=w439) -> ("Arbitrary Feedforward"=w438:dbl)  [unwired: 9 in]
                          n153 = call <vilib>:"SPARK Set Output Advanced.vi"("Arbitrary Feed Forward (0)"=w438, "Control Mode"=Spark_MAX_Control_Type."Percent VBus", "Setpoint"=w439, "MotorControlDevRef"=w441) -> ("error out"=w443:errorcluster, "MotorControlDevRef"=w442:T11)  [unwired: 6 in]
                          n154 = Wait (ms)(milliseconds to wait=u32 500) -> ()  [unwired: 1 out]
                        }
                        n155 = call "Arbitrary Feed Forward Generator.vi"("Feed Forward Constants"=w427, "Setpoint"=w429) -> ("Arbitrary Feedforward"=w430:dbl)  [unwired: 9 in]
                        n156 = call <vilib>:"SPARK Set Sensor Position.vi"("error in"=w436, "Position"=0.0, "MotorControlDeviceRef"=w435) -> ("MotorControlDeviceRef"=w432:T11)  [unwired: 7 in, 1 out]
                        n157 = call <vilib>:"SPARK Set Output Advanced.vi"("Arbitrary Feed Forward (0)"=w430, "Control Mode"=Spark_MAX_Control_Type."Percent VBus", "Setpoint"=w429, "MotorControlDevRef"=w432) -> ()  [unwired: 6 in, 2 out]
                      }
                      frame Disabled {
                      }
                    }
                  }
                  frame Enabled {
                    n158 = call <vilib>:"SPARK Set Output Advanced.vi"("Control Mode"=Spark_MAX_Control_Type."Percent VBus", "Setpoint"=0.0, "MotorControlDevRef"=w446) -> ("MotorControlDevRef"=w445:T11)  [unwired: 7 in, 1 out]
                  }
                }
              }
              frame True {
                n159 = disable-structure shown="Enabled" {
                  disable-tunnel: w461 -> [w490 w511]
                  disable-tunnel: [w484 w513] -> w460
                  disable-tunnel: w459 -> [_ _]
                  disable-tunnel: w458 -> [_ _]
                  disable-tunnel: [w485 w512] -> w456
                  disable-tunnel: w457 -> [w483 w510]
                  disable-tunnel: w455 -> [w488 w508]
                  disable-tunnel: [w489 w507] -> w452
                  disable-tunnel: w454 -> [w487 _]
                  disable-tunnel: w453 -> [w486 _]
                  disable-tunnel: w451 -> [w482 _]
                  disable-tunnel: [w481 _] -> w449
                  frame Enabled {
                    n160 = case shown="False" w482 {
                      tunnel: w490 -> [w499 w504]
                      tunnel: [w498 w501] -> w489
                      tunnel: w488 -> [w497 w503]
                      tunnel: w487 -> [w496 _]
                      tunnel: w486 -> [w495 _]
                      tunnel: [w492 w502] -> w485
                      tunnel: [w494 w500] -> w484
                      tunnel: w483 -> [_ w505]
                      tunnel: [w491 _] -> w481
                      frame False {
                        n161 = call "Trapezoid on the Fly.vi"("FeedForward Constants"=w497, "Setpoint"=0.0, "Acceleration Max"=w495, "Velocity Max"=w496, "MotorControlDevRef in"=w499) -> ("End Time"=w491:dbl, "Sensor Position"=w494:dbl, "MotorControlDevRef out"=w498:T11, "charted V"=w492:cluster{"Sensor Velocity":dbl, "Numeric":dbl}[])  [unwired: 1 out]
                      }
                      frame True {
                        n162 = Negate(x=w505) -> (-x=w506:dbl[])
                        n163 = call "Apply Trapezoid.vi"("FeedForward Constants"=w503, "Velocity values"=w506, "MotorControlDeviceRef in"=w504) -> ("Sensor Position"=w500:dbl, "MotorControlDevRef out"=w501:T11, "charted V"=w502:cluster{"Sensor Velocity":dbl, "Numeric":dbl}[])  [unwired: 5 in, 1 out]
                      }
                    }
                  }
                  frame Disabled {
                    n164 = Negate(x=w510) -> (-x=w509:dbl[])
                    n165 = call "Apply Trapezoid.vi"("FeedForward Constants"=w508, "Velocity values"=w509, "MotorControlDeviceRef in"=w511) -> ("Sensor Position"=w513:dbl, "MotorControlDevRef out"=w507:T11, "charted V"=w512:cluster{"Sensor Velocity":dbl, "Numeric":dbl}[])  [unwired: 5 in, 1 out]
                  }
                }
                n166 = disable-structure shown="Enabled" {
                  disable-tunnel: w455 -> [w465 _]
                  disable-tunnel: w452 -> [w464 _]
                  disable-tunnel: [w462 _] -> w450
                  frame Enabled {
                    w466 = 0.0 ("Setpoint")
                    n167 = disable-structure shown="Enabled" {
                      disable-tunnel: [w472 w480] -> w463
                      disable-tunnel: w465 -> [w471 _]
                      disable-tunnel: w464 -> [w469 w480]
                      frame Disabled {
                        n168 = for {
                          N: 1 -> [_]
                          tunnel: w471 -> [w476]
                          shift-right: [w478] -> w472
                          shift-left: w469 -> [w477]
                          w475 = -0.05 ("Setpoint")
                          (unwired) 0.0 ("Position")
                          n169 = call "Arbitrary Feed Forward Generator.vi"("Feed Forward Constants"=w476, "Setpoint"=w475) -> ("Arbitrary Feedforward"=w474:dbl)  [unwired: 9 in]
                          n170 = call <vilib>:"SPARK Set Output Advanced.vi"("Arbitrary Feed Forward (0)"=w474, "Control Mode"=Spark_MAX_Control_Type."Percent VBus", "Setpoint"=w475, "MotorControlDevRef"=w477) -> ("MotorControlDevRef"=w478:T11)  [unwired: 6 in, 1 out]
                          n171 = Wait (ms)(milliseconds to wait=u32 500) -> ()  [unwired: 1 out]
                        }
                      }
                      frame Enabled {
                      }
                    }
                    n172 = call "Arbitrary Feed Forward Generator.vi"("Feed Forward Constants"=w465, "Setpoint"=w466) -> ("Arbitrary Feedforward"=w467:dbl)  [unwired: 9 in]
                    n173 = call <vilib>:"SPARK Set Output Advanced.vi"("Arbitrary Feed Forward (0)"=w467, "Control Mode"=Spark_MAX_Control_Type."Position", "Setpoint"=w466, "MotorControlDevRef"=w463) -> ("MotorControlDevRef"=w462:T11)  [unwired: 6 in, 1 out]
                  }
                  frame Disabled {
                  }
                }
              }
            }
            "Intake Trapezoid Chart" <- w392
            n174 = call-poly <vilib>:"SPARK Get Device Status.vi"("MotorControlDevRef in"=w383) -> ("Current"=w382:dbl)  [unwired: 7 in, 3 out]
            n175 = disable-structure shown="Enabled" {
              disable-tunnel: "intake setpoint" -> [w525 w578]
              disable-tunnel: w417 -> [w530 w583]
              disable-tunnel: "detected speed (0)" -> [w529 _]
              disable-tunnel: w413 -> [w528 w582]
              disable-tunnel: [w527 _] -> w412
              disable-tunnel: w411 -> [w526 _]
              disable-tunnel: _ -> [_ w581]
              disable-tunnel: Spark_MAX_Control_Type."Percent VBus" ("Control Mode") -> [_ w579]
              disable-tunnel: w396 -> [w517 _]
              disable-tunnel: "launcher speed" -> [w522 _]
              disable-tunnel: w401 -> [w521 _]
              disable-tunnel: [w520 _] -> w400
              disable-tunnel: [w514 _] -> w395
              disable-tunnel: [w516 _] -> w394
              disable-tunnel: [w515 _] -> w384
              disable-tunnel: [w514 _] -> _
              frame Enabled {
                # "cascade lowered?\ntake coral!"
                # "sensed something?\nintake stop (change?)"
                n176 = call "Deadband Checker.vi"("Limit"=0.9 ("upper limit"), "Value"=w517) -> ("Outside Deadband?"=w518:bool)  [unwired: 9 in]
                n177 = Select(t=0.0, s=w518, f=w525) -> (s? t:f=w523:dbl)
                n178 = case shown="False" w521 {
                  tunnel: w530 -> [w534 w569]
                  tunnel: w529 -> [w538 _]
                  tunnel: w528 -> [w541 w567]
                  tunnel: w522 -> [w540 _]
                  tunnel: [w539 TRUE] -> w527
                  tunnel: w526 -> [w537 _]
                  tunnel: w523 -> [w532 w562]
                  tunnel: [w535 1.0] -> w520
                  tunnel: [w533 "sensor speed launcher"] -> w514
                  tunnel: [w532 w562] -> w516
                  tunnel: [w531 w560] -> w515
                  frame False {
                    # "intake"
                    # "intake is set a power"
                    # "just intake no qualms"
                    n179 = case shown="False" w537 {
                      tunnel: w541 -> [w547 w556]
                      tunnel: w540 -> [w544 _]
                      tunnel: [FALSE TRUE] -> w539
                      tunnel: w538 -> [_ w553]
                      tunnel: [5.0 20.0] -> w535
                      tunnel: [w544 w553] -> w533
                      tunnel: [w542 w551] -> w531
                      frame False {
                        # "set norm speed"
                        n180 = disable-structure shown="Enabled" {
                          disable-tunnel: [Spark_MAX_Control_Type."Percent VBus" ("Control Mode") Spark_MAX_Control_Type."Velocity" ("Control Mode")] -> w545
                          frame Disabled {
                          }
                          frame Enabled {
                          }
                        }
                        n181 = call <vilib>:"SPARK Set Output Advanced.vi"("Control Mode"=w545, "Setpoint"=w544, "MotorControlDevRef"=w547) -> ("MotorControlDevRef"=w543:T11)  [unwired: 7 in, 1 out]
                        n182 = call-poly <vilib>:"SPARK Get Encoder Status.vi"("MotorControlDevRef in"=w543) -> ("Sensor Velocity"=w542:dbl)  [unwired: 7 in, 3 out]
                      }
                      frame True {
                        # "todo: previous 1\nexploring cpu usage"
                        # "if it entered the true case set slow 0"
                        # "set launcher to power"
                        n183 = disable-structure shown="Enabled" {
                          disable-tunnel: [Spark_MAX_Control_Type."Percent VBus" ("Control Mode") Spark_MAX_Control_Type."Percent VBus" ("Control Mode")] -> w557
                          frame Enabled {
                          }
                          frame Disabled {
                          }
                        }
                        n184 = call <vilib>:"SPARK Set Output Advanced.vi"("Control Mode"=w557, "Setpoint"=w553, "MotorControlDevRef"=w556) -> ("MotorControlDevRef"=w552:T11)  [unwired: 7 in, 1 out]
                        n185 = call-poly <vilib>:"SPARK Get Encoder Status.vi"("MotorControlDevRef in"=w552) -> ("Sensor Velocity"=w551:dbl)  [unwired: 7 in, 3 out]
                      }
                    }
                    n186 = call <vilib>:"SPARK Set Output Advanced.vi"("Control Mode"=Spark_MAX_Control_Type."Percent VBus", "Setpoint"=w532, "MotorControlDevRef"=w534) -> ()  [unwired: 7 in, 2 out]
                  }
                  frame True {
                    # "funnel"
                    # "logic for limit switch \nfor launcher"
                    n187 = disable-structure shown="Enabled" {
                      disable-tunnel: w567 -> [w576 w577]
                      disable-tunnel: [w573 w577] -> w566
                      frame Disabled {
                        n188 = call-poly <vilib>:"SPARK Configure Limit Switch.vi"("Enabled? (T)"=TRUE, "Polarity (Normally Open)"=Spark_MAX_Limit_Switch_Polarity."Normally Closed", "MotorControlDeviceRef in"=w576) -> ("MotorControlDeviceRef out"=w573:T11)  [unwired: 7 in, 1 out]
                      }
                      frame Enabled {
                      }
                    }
                    n189 = disable-structure shown="Enabled" {
                      disable-tunnel: [Spark_MAX_Control_Type."Percent VBus" ("Control Mode") Spark_MAX_Control_Type."Velocity" ("Control Mode")] -> w568
                      frame Disabled {
                      }
                      frame Enabled {
                      }
                    }
                    n190 = call <vilib>:"SPARK Set Output Advanced.vi"("Control Mode"=Spark_MAX_Control_Type."Percent VBus", "Setpoint"=w562, "MotorControlDevRef"=w569) -> ()  [unwired: 7 in, 2 out]
                    n191 = call <vilib>:"SPARK Set Output Advanced.vi"("Control Mode"=w568, "Setpoint"="sensor speed launcher", "MotorControlDevRef"=w566) -> ("MotorControlDevRef"=w561:T11)  [unwired: 7 in, 1 out]
                    n192 = call-poly <vilib>:"SPARK Get Encoder Status.vi"("MotorControlDevRef in"=w561) -> ("Sensor Velocity"=w560:dbl)  [unwired: 7 in, 3 out]
                  }
                }
                "detect?" <- w521
              }
              frame Disabled {
                # "for testing purposes no sensor \njust running intake and funnel motors"
                n193 = call <vilib>:"SPARK Set Output Advanced.vi"("Control Mode"=w579, "Setpoint"=w581, "MotorControlDevRef"=w582) -> ()  [unwired: 7 in, 2 out]
                n194 = call <vilib>:"SPARK Set Output Advanced.vi"("Control Mode"=Spark_MAX_Control_Type."Percent VBus", "Setpoint"=w578, "MotorControlDevRef"=w583) -> ()  [unwired: 7 in, 2 out]
              }
            }
            "Velocity Chart for Tuning" <- w384
          }
          frame "Scoring Sequence" {
            w604 = T10 0 items=["Slot 0", "Slot 1", "Slot 2", "Slot 3"] ("Closed Loop Slot")
            w614 = T10 0 items=["Slot 0", "Slot 1", "Slot 2", "Slot 3"] ("Closed Loop Slot")
            # "disconnected F here"
            # "dead logic"
            # "v max"
            # "done at comp: if you do not see anything \nin sensor right now = true"
            # "final"
            # "initial"
            # "set 0"
            # "llin reg to convert between trapezoid"
            # "watch susizoids"
            # "setting launcher\nto 0 just in case"
            # "make sure conversion factor is correct"
            # "get current position. check if we are starting from ground or from a non setpoint state. if it is from ground, use known values.\notherwise generate a new one. then do position control to correct"
            n195 = call <vilib>:"SPARK Set Output Advanced.vi"("Arbitrary Feed Forward (0)"=w588, "Control Mode"=Spark_MAX_Control_Type."Position", "Setpoint"=0.0, "MotorControlDevRef"=w620) -> ()  [unwired: 6 in, 2 out]
            n196 = call <vilib>:"SPARK Set Output Advanced.vi"("Control Mode"=Spark_MAX_Control_Type."Percent VBus", "Setpoint"=0.0, "MotorControlDevRef"=w626) -> ()  [unwired: 7 in, 2 out]
            n197 = call-poly <vilib>:"NT Read Value.vi"("name"="/CU-DB/E.E. Setpoint") -> ("value"=w607:dbl)  [unwired: 8 in, 2 out]
            n198 = call <vilib>:"SPARK Set Output Advanced.vi"("Control Mode"=Spark_MAX_Control_Type."Percent VBus", "Setpoint"=0.0, "MotorControlDevRef"=w629) -> ()  [unwired: 7 in, 2 out]
            n199 = Index Array(array=w612, index #1=w613, index #2=w603) -> (element #1=w631:T23, element #2=w602:T23)
            n200 = Unbundle(w631) -> ("Position Setpoint"=w599:dbl, "Trapezoid"=w601:dbl[])  [unwired: 2 out]
            n201 = Unbundle(w602) -> ("Position Setpoint"=w600:dbl)  [unwired: 3 out]
            n202 = Subtract(x=w599, y=w600) -> (x-y=w598:dbl)
            n203 = call "Trapezoid Position Converter.vi"("Distance"=w598, "Initial Parameter"=enum16{"Position", "Trapezoid Distance"}."Position") -> ("Transformed Distance"=w596:dbl)  [unwired: 9 in]
            n204 = call "Generator.vi"("Distance"=w596, "Velocity Max"=w594, "Acceleration Max"=w595) -> ("Velocity values"=w593:dbl[])  [unwired: 7 in, 1 out]
            n205 = Equal?(x=w613, y=Scoring_Levels."L4") -> (x = y?=w616:bool)
            n206 = Select(t=w604, s=w616, f=w614) -> (s? t:f=w605:T10)
            n207 = call-poly <vilib>:"SPARK Get Encoder Status.vi"("MotorControlDevRef in"=w624) -> ("Sensor Position"=w610:dbl, "MotorControlDevRef out"=w611:T11)  [unwired: 7 in, 2 out]
            n208 = Not(x=w587) -> (.not. x?=w586:bool)
            n209 = case shown="True" TRUE {
              tunnel: w623 -> [_ w644]
              tunnel: w605 -> [_ _]
              tunnel: w611 -> [w635 w649]
              tunnel: w610 -> [w636 w642]
              tunnel: [w636 w647] -> w609
              tunnel: w594 -> [_ w648]
              tunnel: w595 -> [_ w646]
              tunnel: w599 -> [_ w645]
              tunnel: w601 -> [_ w641]
              tunnel: w593 -> [_ w640]
              tunnel: w592 -> [_ w639]
              tunnel: [w632 w638] -> w591
              tunnel: [_ w637] -> w589
              frame False {
                n210 = call <vilib>:"SPARK Set Output Advanced.vi"("Control Mode"=Spark_MAX_Control_Type."Percent VBus", "Setpoint"=0.0, "MotorControlDevRef"=w635) -> ("MotorControlDevRef"=w632:T11)  [unwired: 7 in, 1 out]
              }
              frame True {
                # "positional correction"
                # "-12.381"
                n211 = disable-structure shown="Enabled" {
                  disable-tunnel: w649 -> [w663 _]
                  disable-tunnel: w648 -> [w662 _]
                  disable-tunnel: [w661 _] -> w647
                  disable-tunnel: w646 -> [w660 _]
                  disable-tunnel: w645 -> [w659 _]
                  disable-tunnel: w644 -> [w653 _]
                  disable-tunnel: [w658 _] -> w643
                  disable-tunnel: w642 -> [w656 _]
                  disable-tunnel: w641 -> [w655 _]
                  disable-tunnel: w640 -> [w654 _]
                  disable-tunnel: w639 -> [w652 _]
                  disable-tunnel: [w651 _] -> w638
                  disable-tunnel: [w650 _] -> w637
                  frame Enabled {
                    n212 = case shown="False" w652 {
                      tunnel: w663 -> [w673 w687]
                      tunnel: w662 -> [w672 _]
                      tunnel: [w671 w677] -> w661
                      tunnel: w660 -> [w670 _]
                      tunnel: w659 -> [w669 w675]
                      tunnel: [w667 w688] -> w658
                      tunnel: [w666 w689] -> w657
                      tunnel: w656 -> [_ w686]
                      tunnel: w655 -> [_ w685]
                      tunnel: w654 -> [_ w683]
                      tunnel: w653 -> [w668 w676]
                      tunnel: [w665 w674] -> w651
                      tunnel: [w664 _] -> w650
                      frame False {
                        n213 = call "Trapezoid on the Fly.vi"("FeedForward Constants"=w668, "Setpoint"=w669, "Acceleration Max"=w670, "Velocity Max"=w672, "MotorControlDevRef in"=w673) -> ("End Time"=w664:dbl, "Post-Trapezoid Sensor Position"=w667:dbl, "Sensor Position"=w671:dbl, "MotorControlDevRef out"=w665:T11, "charted V"=w666:cluster{"Sensor Velocity":dbl, "Numeric":dbl}[])
                      }
                      frame True {
                        w680 = T10 0 items=["Slot 0", "Slot 1", "Slot 2", "Slot 3"] ("Closed Loop Slot")
                        n214 = call "Deadband Checker.vi"("Limit"=1.5, "Value"=w686) -> ("Outside Deadband?"=w690:bool)  [unwired: 9 in]
                        n215 = Not(x=w690) -> (.not. x?=w692:bool)
                        n216 = Select(t=w685, s=w692, f=w683) -> (s? t:f=w684:dbl[])
                        n217 = call "Apply Trapezoid.vi"("FeedForward Constants"=w676, "Velocity values"=w684, "MotorControlDeviceRef in"=w687) -> ("Sensor Position"=w688:dbl, "MotorControlDevRef out"=w682:T11, "charted V"=w689:cluster{"Sensor Velocity":dbl, "Numeric":dbl}[])  [unwired: 5 in, 1 out]
                        n218 = call "Arbitrary Feed Forward Generator.vi"("Feed Forward Constants"=w676, "Setpoint"=w675) -> ("Arbitrary Feedforward"=w681:dbl)  [unwired: 9 in]
                        n219 = call <vilib>:"SPARK Set Output Advanced.vi"("Arbitrary Feed Forward (0)"=w681, "Closed Loop Slot"=w680, "Control Mode"=Spark_MAX_Control_Type."Position", "Setpoint"=w675, "MotorControlDevRef"=w682) -> ("MotorControlDevRef"=w678:T11)  [unwired: 5 in, 1 out]
                        n220 = call-poly <vilib>:"SPARK Get Encoder Status.vi"("MotorControlDevRef in"=w678) -> ("Sensor Position"=w677:dbl, "MotorControlDevRef out"=w674:T11)  [unwired: 7 in, 2 out]
                      }
                    }
                    "Scoring Sequence Trapezoid" <- w657
                  }
                  frame Disabled {
                    w700 = T10 0 items=["Slot 0", "Slot 1", "Slot 2", "Slot 3"] ("Closed Loop Slot")
                    n221 = call "Arbitrary Feed Forward Generator.vi"() -> ("Arbitrary Feedforward"=w694:dbl, "Setpoint"=w693:dbl)  [unwired: 10 in]
                    n222 = call <vilib>:"SPARK Set Output Advanced.vi"("Arbitrary Feed Forward (0)"=w694, "Closed Loop Slot"=w700, "Control Mode"=Spark_MAX_Control_Type."Position", "Setpoint"=w693) -> (3:"MotorControlDevRef"=w698:T11, 11:"MotorControlDevRef"=w701:T11)  [unwired: 5 in, 1 out]
                    n223 = call-poly <vilib>:"SPARK Get Encoder Status.vi"("MotorControlDevRef in"=w698) -> ("Sensor Position"=w696:dbl)  [unwired: 7 in, 3 out]
                    n224 = Bundle("Sensor Position"=w696) -> (w697:cluster{"Sensor Position":dbl, void}, w695)  [unwired: 1 in]
                  }
                }
                "Post-Trapezoid Sensor Position" <- w643
              }
            }
            "Post Position Correction" <- w609
            n225 = call-poly <vilib>:"SPARK Get Device Status.vi"("MotorControlDevRef in"=w591) -> ("Current"=w590:dbl)  [unwired: 7 in, 3 out]
          }
          frame "Score" {
            w720 = T10 0 items=["Slot 0", "Slot 1", "Slot 2", "Slot 3"] ("Closed Loop Slot")
            # "launcher"
            # "coral LAUNCH"
            n226 = Index Array(array=w717, index=w716) -> (element=w715:T23)
            n227 = call "Arbitrary Feed Forward Generator.vi"("Feed Forward Constants"=w721) -> ("Arbitrary Feedforward"=w722:dbl)  [unwired: 10 in]
            n228 = Unbundle(w715) -> ("Position Setpoint"=w713:dbl, "Score Power"=w707:dbl)  [unwired: 2 out]
            n229 = call <vilib>:"SPARK Set Output Advanced.vi"("Arbitrary Feed Forward (0)"=w722, "Closed Loop Slot"=w720, "Control Mode"=Spark_MAX_Control_Type."Position", "Setpoint"=w713, "MotorControlDevRef"=w714) -> ("MotorControlDevRef"=w712:T11)  [unwired: 5 in, 1 out]
            n230 = call-poly <vilib>:"SPARK Get Encoder Status.vi"("MotorControlDevRef in"=w712) -> ("Sensor Position"=w708:dbl, "MotorControlDevRef out"=w703:T11)  [unwired: 7 in, 2 out]
            n231 = call <vilib>:"SPARK Set Output Advanced.vi"("Control Mode"=Spark_MAX_Control_Type."Percent VBus", "Setpoint"=w707, "MotorControlDevRef"=w711) -> ()  [unwired: 7 in, 2 out]
            n232 = call-poly <vilib>:"SPARK Get Device Status.vi"("MotorControlDevRef in"=w703) -> ("Current"=w702:dbl)  [unwired: 7 in, 3 out]
            n233 = call-poly <vilib>:"NT Read Value.vi"("name"="/CU-DB/Intake Setpoint") -> ("value"=w705:dbl)  [unwired: 8 in, 2 out]
          }
          frame "Manual Override" {
            w734 = 0.2 ("t")
            # "set power to control cascade"
            n234 = Negate(x=w734) -> (-x=w733:dbl)
            n235 = Select(t=w733, s=w744, f=w734) -> (s? t:f=w740:dbl)
            n236 = call "Arbitrary Feed Forward Generator.vi"("Feed Forward Constants"=w741, "Setpoint"=w740) -> ("Arbitrary Feedforward"=w742:dbl)  [unwired: 9 in]
            n237 = call <vilib>:"SPARK Set Output Advanced.vi"("Arbitrary Feed Forward (0)"=w742, "Control Mode"=Spark_MAX_Control_Type."Percent VBus", "Setpoint"=w740, "MotorControlDevRef"=w745) -> ("MotorControlDevRef"=w736:T11)  [unwired: 6 in, 1 out]
            n238 = call-poly <vilib>:"SPARK Get Encoder Status.vi"("MotorControlDevRef in"=w736) -> ("Sensor Position"=w732:dbl, "MotorControlDevRef out"=w726:T11)  [unwired: 7 in, 2 out]
            n239 = call-poly <vilib>:"SPARK Get Device Status.vi"("MotorControlDevRef in"=w726) -> ("Current"=w725:dbl)  [unwired: 7 in, 3 out]
            n240 = call-poly <vilib>:"NT Read Value.vi"("name"="/CU-DB/Intake Setpoint") -> ("value"=w728:dbl)  [unwired: 8 in, 2 out]
            n241 = call-poly <vilib>:"NT Read Value.vi"("name"="/CU-DB/E.E. Setpoint") -> ("value"=w730:dbl)  [unwired: 8 in, 2 out]
          }
          frame "Hold Position" {
            w747 = T10 0 items=["Slot 0", "Slot 1", "Slot 2", "Slot 3"] ("Closed Loop Slot")
            w775 = T10 0 items=["Slot 0", "Slot 1", "Slot 2", "Slot 3"] ("Closed Loop Slot")
            # "this should be false"
            # "cascade"
            # "suspect"
            # "hold whatever positon you are at after manual override or scoring sequence"
            n242 = Index Array(array=w765, index=w764) -> (element=w763:T23)
            n243 = Unbundle(w763) -> ("Position Setpoint"=w762:dbl)  [unwired: 3 out]
            n244 = Not(x=w754) -> (.not. x?=w753:bool)
            n245 = And(x=w753, y=w752) -> ()  [unwired: 1 out]
            n246 = call-poly <vilib>:"SPARK Get Encoder Status.vi"("MotorControlDevRef in"=w778) -> ("Sensor Position"=w774:dbl, "MotorControlDevRef out"=w773:T11)  [unwired: 7 in, 2 out]
            n247 = call <vilib>:"SPARK Set Output Advanced.vi"("Arbitrary Feed Forward (0)"=w748, "Closed Loop Slot"=w775, "Control Mode"=Spark_MAX_Control_Type."Position", "Setpoint"=w774, "MotorControlDevRef"=w773) -> ()  [unwired: 5 in, 2 out]
            n248 = call "Arbitrary Feed Forward Generator.vi"("Feed Forward Constants"=w776, "Setpoint"=w774) -> ("Arbitrary Feedforward"=w768:dbl)  [unwired: 9 in]
            n249 = Equal?(x=Scoring_Levels."L4" ("y"), y=w764) -> (x = y?=w769:bool)
            n250 = Select(t="L4 Increased FF", s=w769, f=w768) -> (s? t:f=w766:dbl)
            n251 = call-poly <vilib>:"SPARK Get Encoder Status.vi"("MotorControlDevRef in"=w779) -> ("Sensor Position"=w759:dbl, "MotorControlDevRef out"=w780:T11)  [unwired: 7 in, 2 out]
            n252 = call <vilib>:"SPARK Set Output Advanced.vi"("Arbitrary Feed Forward (0)"=w766, "Closed Loop Slot"=w747, "Control Mode"=Spark_MAX_Control_Type."Position", "Setpoint"=w762, "MotorControlDevRef"=w780) -> ("MotorControlDevRef"=w750:T11)  [unwired: 5 in, 1 out]
            n253 = call-poly <vilib>:"SPARK Get Device Status.vi"("MotorControlDevRef in"=w750) -> ("Current"=w749:dbl)  [unwired: 7 in, 3 out]
            n254 = call-poly <vilib>:"NT Read Value.vi"("name"="/CU-DB/E.E. Setpoint") -> ("value"=w757:dbl)  [unwired: 8 in, 2 out]
            n255 = call-poly <vilib>:"NT Read Value.vi"("name"="/CU-DB/Intake Setpoint") -> ("value"=w755:dbl)  [unwired: 8 in, 2 out]
          }
        }
        "Current" <- w176
        "End Time" <- w175
        n256 = feedback-in #5(w181) -> ()
        n257 = feedback-in #6(w202) -> ()
        n258 = Bundle("Sensor Position"=w197) -> (→"Position Chart (All Time)":cluster{"Sensor Position":dbl})  [unwired: 1 in]
        n259 = global write "Robot Global Data.vi" "Can Climb?"(w203) -> ()
        n260 = call-poly <vilib>:"NT Write Value.vi"("value"=w187, "name"="/CU-DB/Cascade Sensor") -> ()  [unwired: 9 in, 1 out]
        n261 = call-poly <vilib>:"NT Write Value.vi"("value"=w186, "name"="/CU-DB/E.E. Setpoint") -> ()  [unwired: 9 in, 1 out]
        n262 = call-poly <vilib>:"NT Write Value.vi"("value"=w183, "name"="/CU-DB/Intake Setpoint") -> ()  [unwired: 9 in, 1 out]
      }
      frame "Calibrate" {
        # "set cascade/pivot to 0"
        n263 = call <vilib>:"SPARK Set Output Advanced.vi"("Control Mode"=Spark_MAX_Control_Type."Percent VBus", "Setpoint"=0.0, "MotorControlDevRef"=w786) -> ()  [unwired: 7 in, 2 out]
        n264 = call <vilib>:"SPARK Set Output Advanced.vi"("Control Mode"=Spark_MAX_Control_Type."Percent VBus", "Setpoint"=0.0, "MotorControlDevRef"=w783) -> ()  [unwired: 7 in, 2 out]
        n265 = call <vilib>:"SPARK Set Sensor Position.vi"("Position"=0.0, "MotorControlDeviceRef"=w792) -> ()  [unwired: 8 in, 2 out]
        n266 = call <vilib>:"SPARK Set Sensor Position.vi"("Position"=0.0, "MotorControlDeviceRef"=w787) -> ()  [unwired: 8 in, 2 out]
      }
      frame "Reserve" {
        w808 = -1.0  # Infinite
        # "because it foundationally does the same thing as reserve"
        # "set comment or print to say you should NOT want to be in here"
        # "If loop needs to poll sensors or other\nvalues, use a timeout value. -1 waits for\nnext command to be sent."
        n267 = call-poly <vilib>:"SPARK Get Encoder Status.vi"("MotorControlDevRef in"=w803) -> ("Sensor Position"=w804:dbl, "MotorControlDevRef out"=w805:T11)  [unwired: 7 in, 2 out]
        n268 = call-poly <vilib>:"SPARK Get Encoder Status.vi"("MotorControlDevRef in"=w793) -> ("Sensor Position"=w794:dbl, "MotorControlDevRef out"=w795:T11)  [unwired: 7 in, 2 out]
        n269 = call <vilib>:"SPARK Set Output Advanced.vi"("Control Mode"=Spark_MAX_Control_Type."Percent VBus", "Setpoint"=0.0, "MotorControlDevRef"=w802) -> ()  [unwired: 7 in, 2 out]
        n270 = call <vilib>:"SPARK Set Output Advanced.vi"("Control Mode"=Spark_MAX_Control_Type."Position", "Setpoint"=w804, "MotorControlDevRef"=w805) -> ()  [unwired: 7 in, 2 out]
        n271 = call <vilib>:"SPARK Set Output Advanced.vi"("Control Mode"=Spark_MAX_Control_Type."Position", "Setpoint"=w794, "MotorControlDevRef"=w795) -> ()  [unwired: 7 in, 2 out]
        n272 = call <vilib>:"SPARK Set Output Advanced.vi"("Control Mode"=Spark_MAX_Control_Type."Percent VBus", "Setpoint"=0.0, "MotorControlDevRef"=w797) -> ()  [unwired: 7 in, 2 out]
      }
    }
    n273 = call "Coral Check for New Command.vi"("Current Command"=w140, "Wait time (ms)"=w145, "Finished?"=w146) -> ("Completion"=w141:T7, "Subsystem Name"=w142:string, "Current Command"=w143:T3, "Initial Trace String"=w144:string, "NextCommand"=w147:T18)  [unwired: 4 in]
    n274 = case shown="\"Successful\", \"Aborted\"" w141 {
      selector: w141 -> [_ w816]
      tunnel: w144 -> [_ w812]
      tunnel: w143 -> [_ w813]
      tunnel: w142 -> [_ w809]
      frame "Incomplete", Default {
        # "Continuing current command"
      }
      frame "Successful", "Aborted" {
        # "Report and setup for next command"
        n275 = Unbundle By Name(w813) -> ("Coral States"=w815:T5, "Setpoint State"=w810:T6)
        n276 = Format Into String(format string="CS %s, SS %s", initial string=w812, w815, w810) -> (resulting string=w811:string)  [unwired: 1 in, 1 out]
        "Current\nCmd" <- w811
        n277 = call <vilib>:"Trace Results.vi"("Status of previous command"=w816, "Description"=w811, "Subsystem"=w809) -> ()  [unwired: 9 in]
      }
    }
    n278 = disable-structure shown="Enabled" {
      frame Disabled {
        # "Publish"
        n279 = call-poly <vilib>:"NT Write Value.vi"() -> ()  [unwired: 11 in, 1 out]
      }
      frame Enabled {
      }
    }
  }
